vi "GTcode_v6(reorganized).vi"() -> ()   [LabVIEW 2016]
uses:
  DCScode_simulISS_MAP/flex05-4chPascal.dll
  <vilib>/Utility/config.llb/NI_LVConfig.lvlib
  <vilib>/Utility/config.llb/Write Key (U32).vi
  <vilib>/Utility/config.llb/Read Key (U32).vi
  DCScode_simulISS_MAP/flex05oem8chauto100nsPASCAL_win7.dll
  <vilib>/Analysis/NI_AALBase.lvlib
  <vilib>/Analysis/NI_AALPro.lvlib
  <vilib>/Utility/config.llb/Write Key (I32).vi
  <vilib>/Utility/config.llb/Write Key (Double).vi
  <vilib>/Utility/config.llb/Write Key (String).vi
  <vilib>/Utility/config.llb/Read Key (I32).vi
  <vilib>/Waveform/WDTOps.llb/WDT Append Waveforms DBL.vi
  <vilib>/Waveform/WDTFileIO.llb/ Write Waveform to File.vi
  <vilib>/Analysis/5stat.llb/RMS (DBL).vi
panel:
  in  "Tab\nControl":T1(tab)=enum."Real Time Fitting Parameters" caption="Tab Control"
  out "mean":dbl format="%0.1e"
  out "COV":dbl format="%0.1f"
  in  "Fixed Time":bool
  in  "Detector Used":T2(ring)=enum."Det 2"
  in  "Real Time Fitting?":bool=TRUE
  out "g2":cluster{"Delay Time":sgl[], sgl[]}[](graph) caption="Normalized Correlation Function"
  out "Tau":cluster{"tmp":dbl, dbl}(graph) caption="Relative Changes of Flow"
  in  "QUIT":bool
  in  "Clear plots":bool
  in  "Baseline":bool
  in  "MARK\nMark":bool
  in  "Stop":bool
  in  "Sequence Scan":bool
  out "Mark #":u32
  out "Trial #":u32
  out "Frame #":u32
  out "Det 8":sgl format="%.3f"
  out "Det 7":sgl format="%.3f"
  out "Det 6":sgl format="%.3f"
  out "Det 5":sgl format="%.3f"
  out "Det 4":sgl format="%.3f"
  out "Det 3":sgl format="%.3f"
  out "Det 2":sgl format="%.3f"
  out "Det 1":sgl format="%.3f"
  out "Computer Time":string="2010-1-12 23:16:10"
  in  "D1":bool
  in  "D2":bool
  in  "D3":bool
  in  "D4":bool
  in  "D5":bool
  in  "D6":bool
  in  "D7":bool
  in  "D8":bool
  out "Tau 2":T3(graph)={1.6593152555505744e-08, 3.9427894777554196e-08, 4.065716407938411e-08, 1.5135790977358522e-08, 2.4870420100428357e-08, 7.094765128107397e-08, 0.0, 4.1348620928852906e-07, 1.5886917674344795e-08, 4.0280526032721455e-08, -1.0, -1.0} caption="Blood Flow Index (cm2/s)"
  in  "Fixed # of Frames":u32=5
  out "Status":string="Quit"
  in  "Optical Switch OPEN":bool
  in  "Delay between frames(ms)":u32=500
  out "Time Left (ms)":sgl format="%.3f"
  in  "Integration Time (ms)":sgl=1000.0 min=1 max=13000 step=1
  in  "File Name:":string="test0"
  in  "Data Save Directory:":path=path "C:/data"
  in  "ISS Lasers ON":bool
  in  "Test":bool
  out "Moving Avg RMS":dbl(slide) scale=0.0..0.07
  out "raw data":dynamicdata(graph)
  out "Trial Data 2":waveform(dbl)(graph)
  out "Moving Avg RMS Graph":dbl(graph)
  out "Reset Data Acquisition\nAnd UI Updating":bool=TRUE
  out "Trial In Progress":bool
  in  "Lines":tag="Dev1/port1/line0:1, Dev1/port1/line3:7"
  in  "Delaytime(ms)":u32=200
  in  "Initialize Correlator":bool
  in  "Detector Select":enum32{"4 Detectors", "8 Detectors"}(radio)=enum."8 Detectors"
  in  "Update Time (ms)\nDO NOT CHANGE!":u32=105 min=1 max=999 step=1
  in  "Laser Input Name":refnum<visa-resource-name>="COM7"
  out "Flow in each detector":dbl[](array[numeric])=[-1.0, -1.0, -1.0, -1.0, -1.0, -1.0, -1.0, -1.0, -1.0, -1.0, -1.0, -1.0]
  in  "Visible\nAverages":bool[](array[boolean])=[FALSE, FALSE, FALSE, FALSE]
  in  "Avg":bool[][](array[boolean])=[[FALSE, FALSE, FALSE, FALSE, FALSE, FALSE, FALSE, FALSE], [FALSE, FALSE, FALSE, FALSE, FALSE, FALSE, FALSE, FALSE], [FALSE, FALSE, FALSE, FALSE, FALSE, FALSE, FALSE, FALSE], [FALSE, FALSE, FALSE, FALSE, FALSE, FALSE, FALSE, FALSE]]
  in  "rho":dbl[](array[numeric])=[2.5, 2.5, 2.5, 2.5, 2.5, 2.5, 2.5, 2.5, -1.0, -1.0, -1.0, -1.0]
  in  "Other Settings":u32[](array[numeric])=[1, 120, 0, 1] caption="Flow in each detector"
  in  "Initial Guess":dbl[](array[numeric])=[1e-08, 0.5, 0.05, 10.0] caption="Flow in each detector"
  in  "Lower Cut-Off":dbl=20.0
  in  "Upper Cut-Off (Not In Use)":dbl=300.0 caption="Upper Cut-Off"
  in  "Sample rate (Hz)":dbl=22050.0
  in  "Frames Per Second":dbl
  in  "Moving Average Length (s)":dbl
  in  "VR Data Input File":path
  in  "VR Percent Path":path
  out "Bufffer Index":dbl
  out "Frames in Buffer":dbl
  out "Samples per frame":dbl
  out "Filtered data":waveform(dbl)
  out "Rectified Moving Average Sample":waveform(dbl)[](graph)
  out "Trial Data":waveform(dbl)
  in  "Trial Number":dbl
  in  "Target Percentage":dbl
  out "Aggregate Data":waveform(dbl)[](array[waveform])
  out "4CH?":bool
  out "Detector#":u32=1
  out "Source#":u32=1
  # "kHz"
  # "kHz"
  # "Don't Change these Parameters unless you know clearly what you are doing"
  # "ISS Triggers Setup"
  # "Channel Parameters"
  # "Step1"
  # "Line"
  # "0"
  # "1"
  # "3"
  # "4"
  # "5"
  # "6"
  # "7"
  # "*The number of lines in the list must\nmatch the number of elements in\nthe array."
  # "Step2"
  # "Line"
  # "0"
  # "1"
  # "3"
  # "4"
  # "5"
  # "6"
  # "7"
  # "Step3"
  # "Line"
  # "0"
  # "1"
  # "3"
  # "4"
  # "5"
  # "6"
  # "7"
  # "Line    Signal\n\n0           ISS Trigger (0: OFF, 1: ON)\n1           Flow Laser 1 ON/OFF (0:OFF, 1:ON)\n2           ISS Data Acquisition (0: DONE, 1: NO)\n3           ISS Laser ON/OFF (0: ON, 1: OFF)\n4           Trigger for Marks  (0: OFF, 1: ON)\n5           Flow Laser 2 ON/OFF (0:OFF, 1:ON)\n6           Reserved\n7           Reserved"
  # "Wait ISS Data Acuisition DONE Signal"
  # "Step4"
  # "Step5"
  # "Line"
  # "0"
  # "1"
  # "3"
  # "4"
  # "5"
  # "6"
  # "7"
  # "Flow Lasers Setup"
  # "FROM FRONT PANEL"
  # "Line"
  # "0"
  # "1"
  # "3"
  # "4"
  # "5"
  # "6"
  # "7"
  # "Line"
  # "0"
  # "1"
  # "3"
  # "4"
  # "5"
  # "6"
  # "7"
  # "Det 1"
  # "Det 2"
  # "Det 3"
  # "Det 4"
  # "Det 5"
  # "Det 6"
  # "Det 7"
  # "Det 8"
  # "Avg 1"
  # "Avg 2"
  # "Avg 3"
  # "Avg 4"
  # "Db"
  # "Beta"
  # "Mua"
  # "MuS'"
  # "1"
  # "2"
  # "3"
  # "4"
  # "5"
  # "6"
  # "7"
  # "8"
  # "Avg 1"
  # "Starting Pt"
  # "End Pt"
  # "Approximate"
  # "Variables"
  # "Avg 2"
  # "Avg 3"
  # "Avg 4"
  # "Source Detector  Separations"
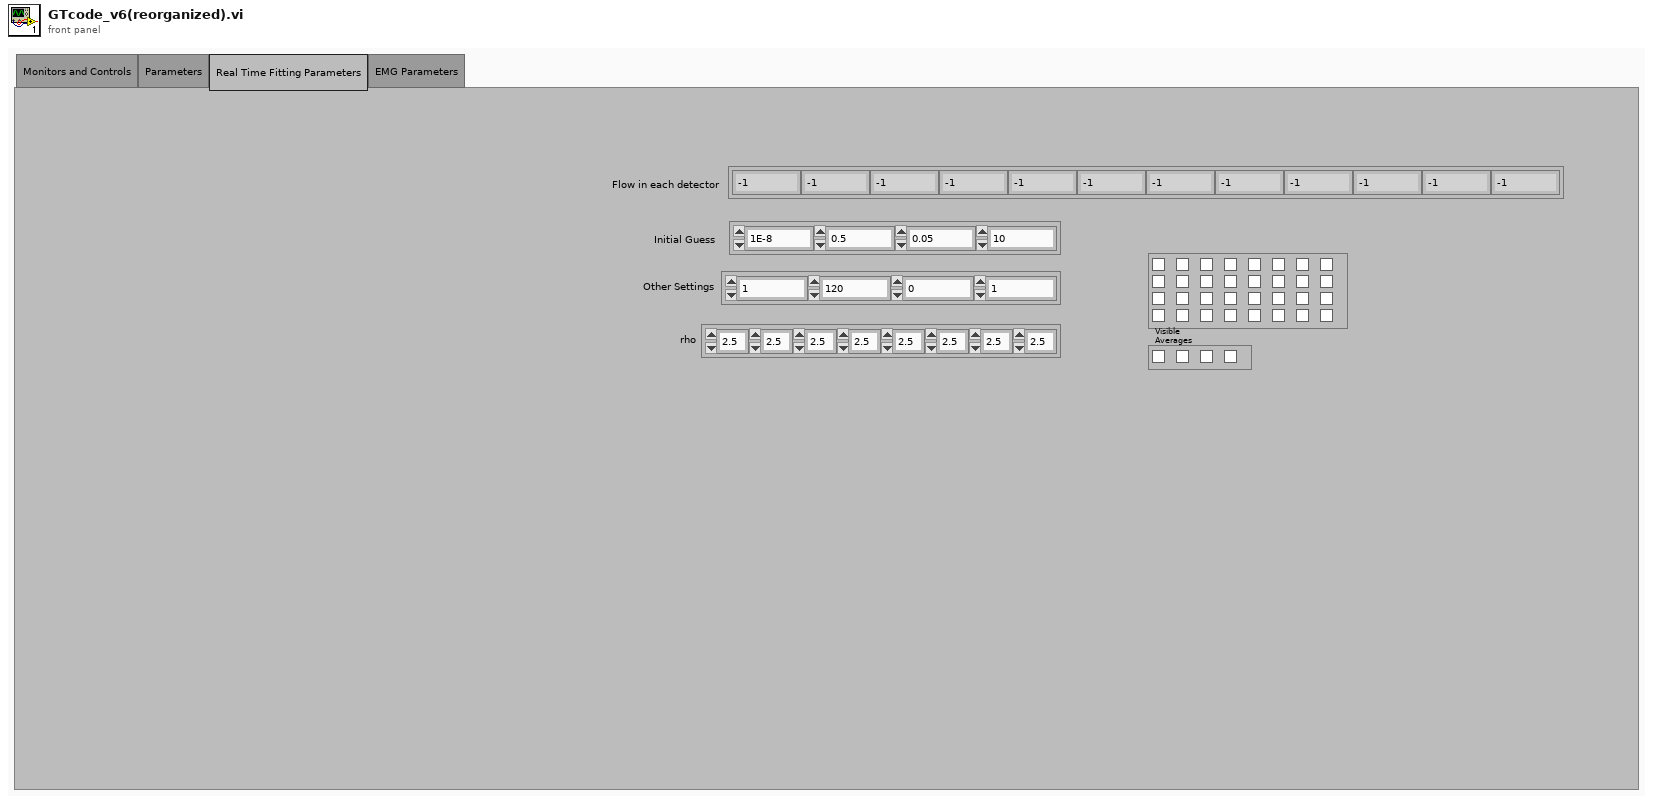
[diagram p1: front panel]
types:
  T1 = enum32{"Monitors and Controls", "Parameters", "Real Time Fitting Parameters", "EMG Parameters"}
  T2 = enum16{"Det 1", "Det 2", "Det 3", "Det 4", "Det 5", "Det 6", "Det 7", "Det 8"}
  T3 = cluster{dbl, dbl, dbl, dbl, dbl, dbl, dbl, dbl, dbl, dbl, dbl, dbl}
  T4 = typedef "WaveformArrayControl.ctl" = waveform(dbl)[]
  T5 = enum8{"Enabled", "Disabled", "Disabled and Grayed Out"}
  T6 = cluster{dbl, dbl, dbl, dbl, dbl, dbl, dbl, dbl, dbl, dbl, dbl, dbl}[]
  T7 = typedef "NI_LVConfig.lvlib/Config Data RefNum.ctl" = refnum<k1>
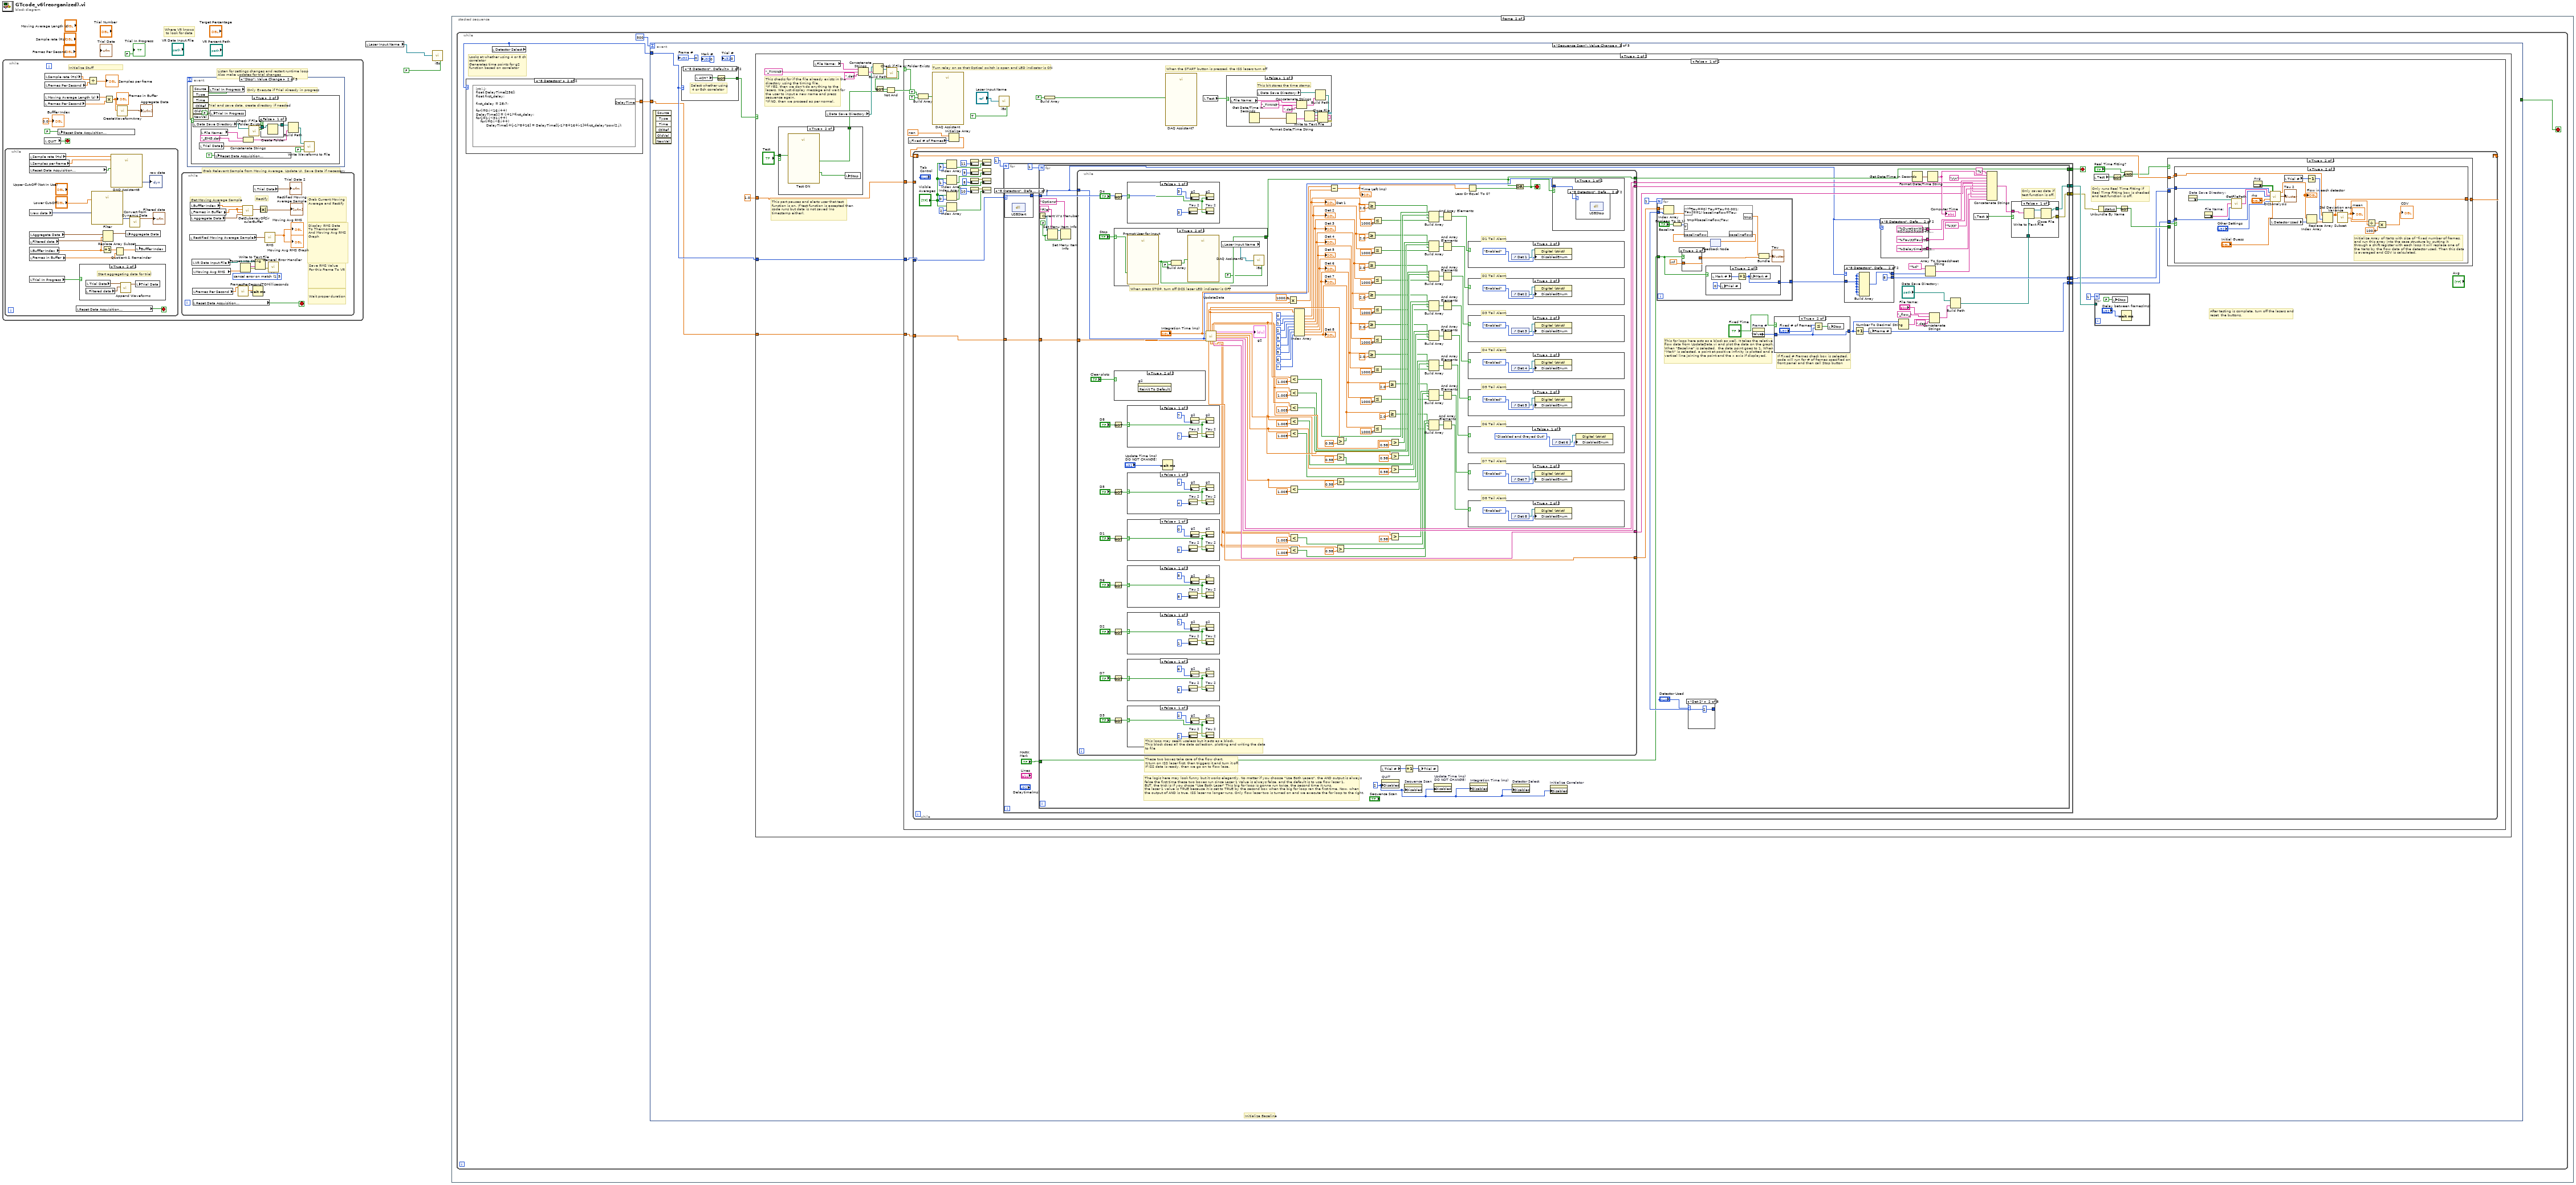
[diagram p0: block diagram]
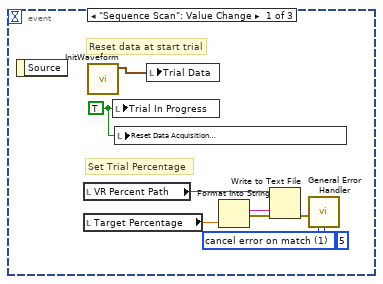
[diagram p2: hidden frame]
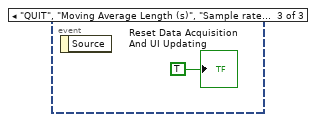
[diagram p5: hidden frame]
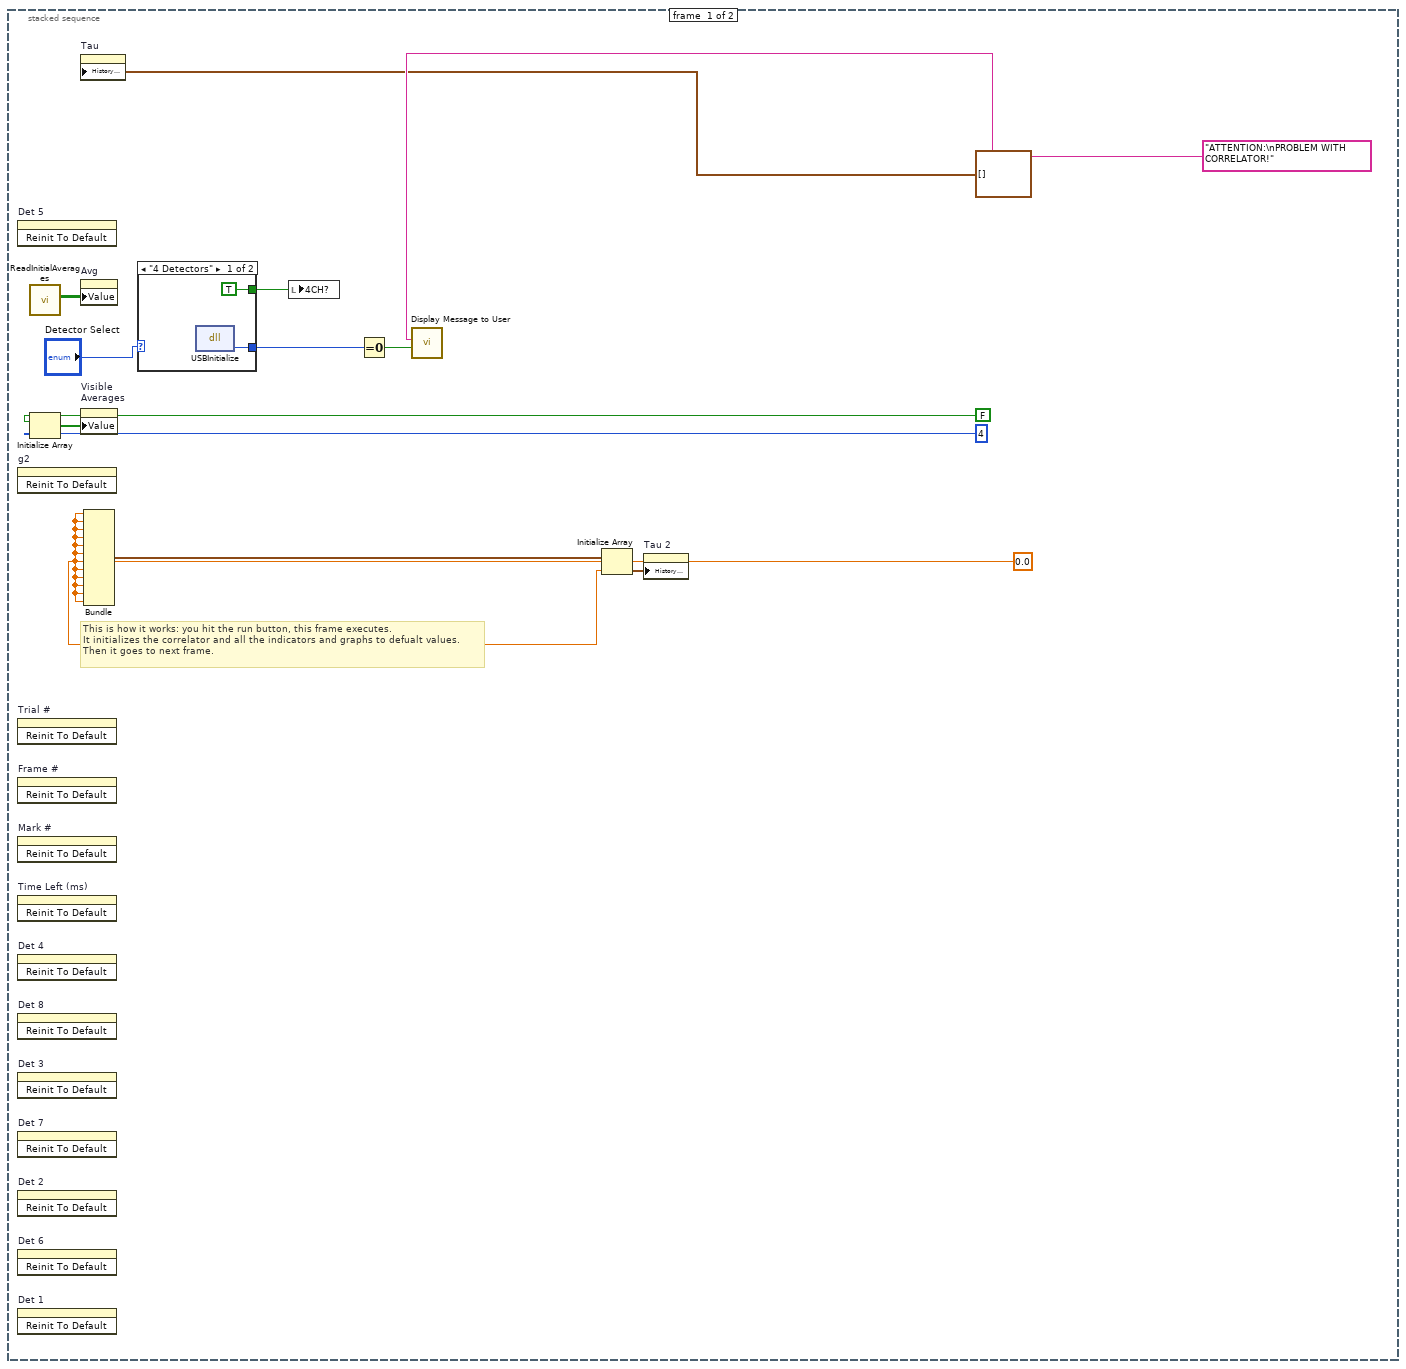
[diagram p7: hidden frame]
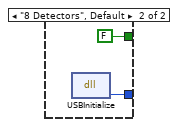
[diagram p8: hidden frame]
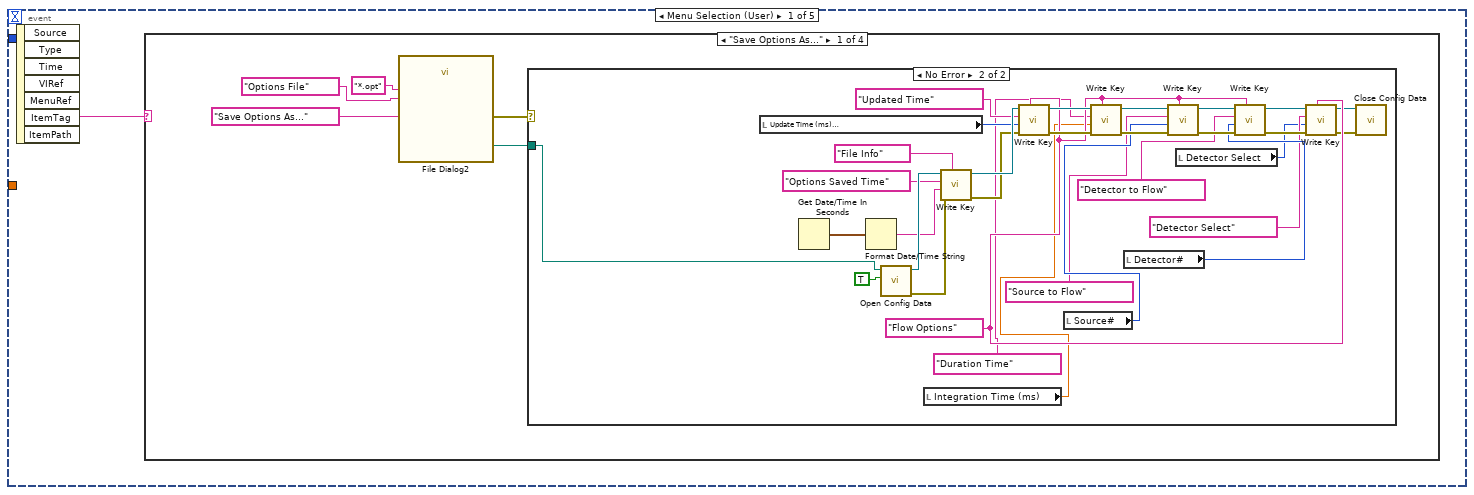
[diagram p10: hidden frame]
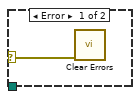
[diagram p11: hidden frame]
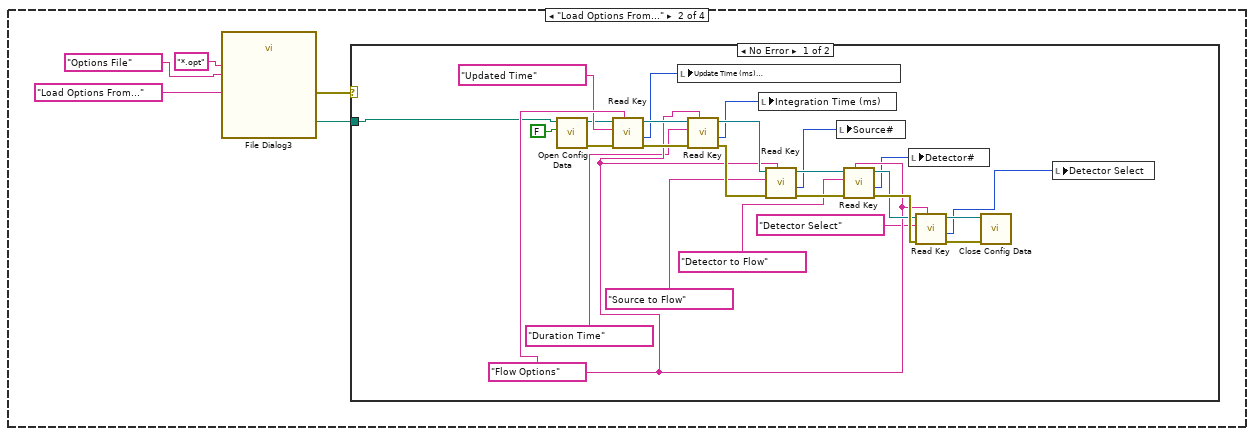
[diagram p12: hidden frame]
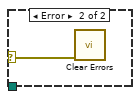
[diagram p13: hidden frame]
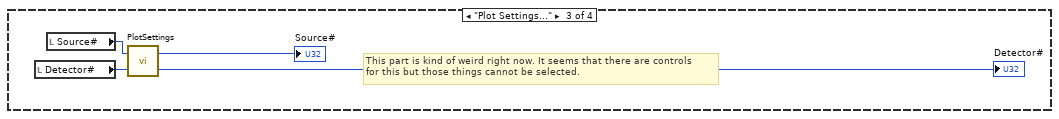
[diagram p14: hidden frame]
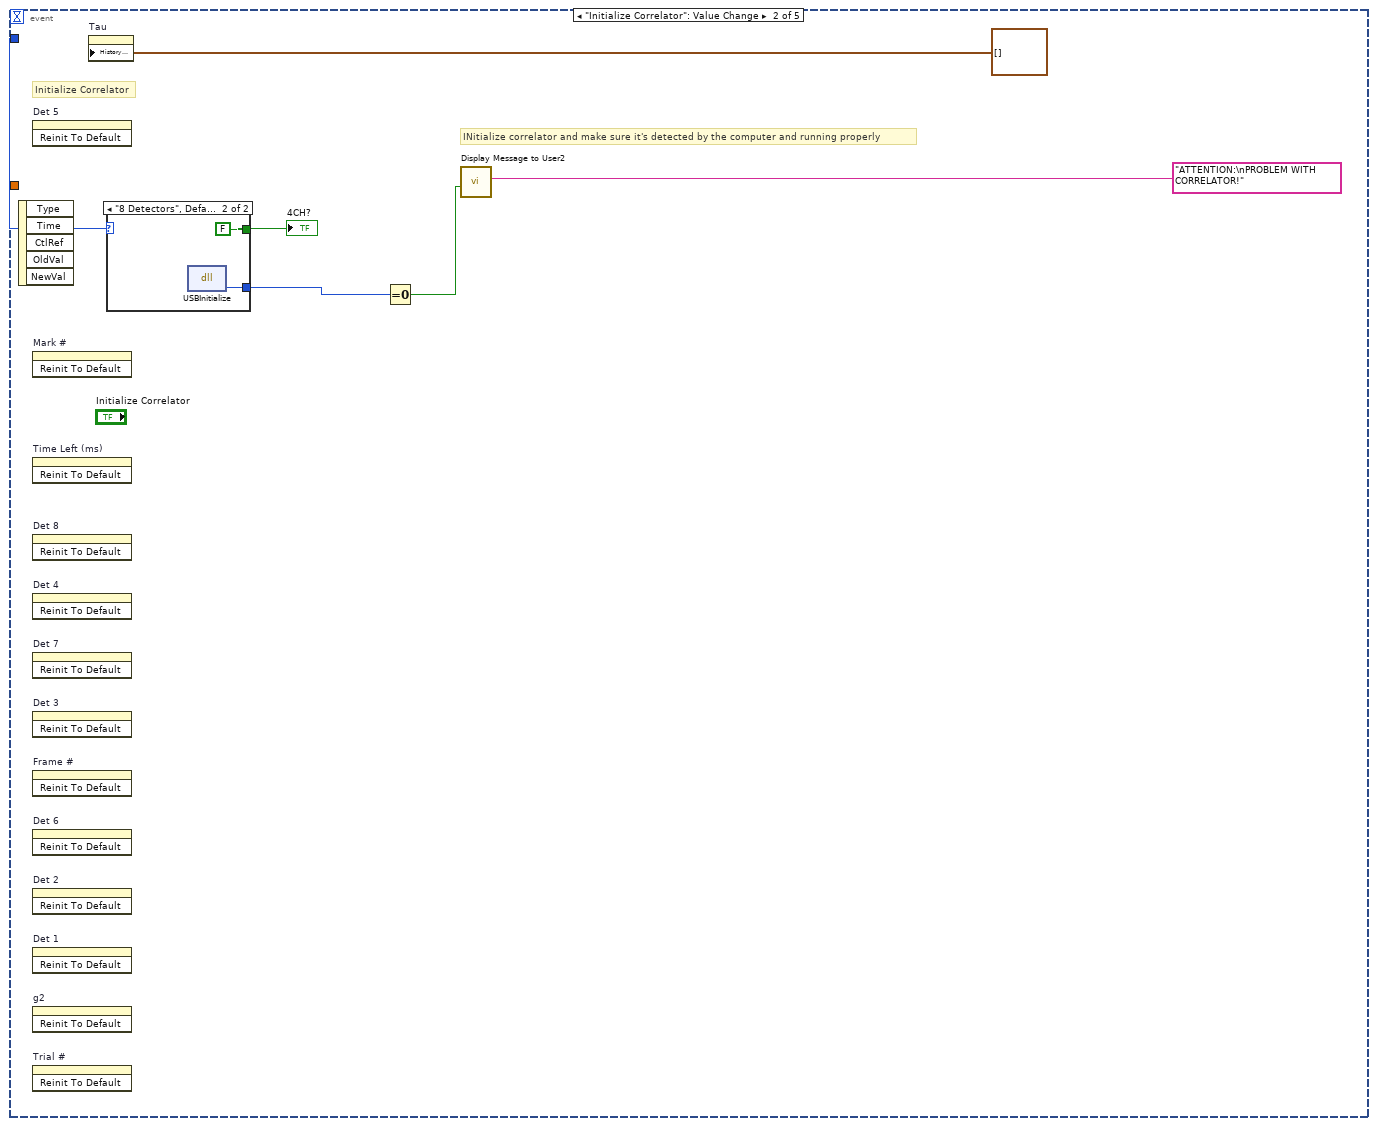
[diagram p16: hidden frame]
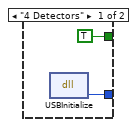
[diagram p17: hidden frame]
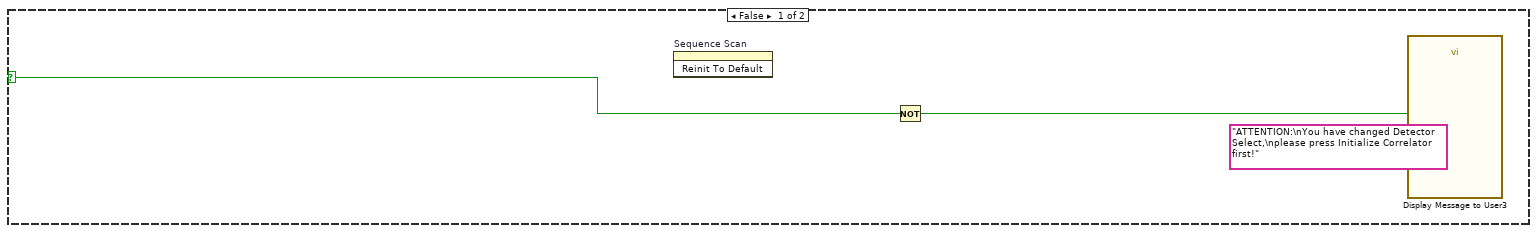
[diagram p18: hidden frame]
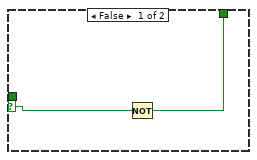
[diagram p19: hidden frame]
diagram:
  # "Where VR knows\n to look for data"
  n1 = while {
    stop <- w4 stop-if-true
    # "Grab Relevant Sample from Moving Average, Update UI, Save Data if necessary"
    # "Initialize Stuff"
    # "Listen for settings changes and restart runtime loop\nAlso make updates for trial changes"
    n2 = while {
      stop <- w60 stop-if-true
      n3 = local read "Sample rate (Hz)"() -> (w74:dbl)
      n4 = local read "Samples per frame"() -> (w73:dbl)
      n5 = local read "Reset Data Acquisition\nAnd UI Updating"() -> (w59:bool)
      n6 = local read "raw data"() -> (w71:dynamicdata)
      n7 = local read "Aggregate Data"() -> (w67:waveform(dbl)[])
      n8 = local read "Filtered data"() -> (w66:waveform(dbl))
      n9 = local read "Bufffer Index"() -> (w65:dbl)
      n10 = local read "Frames in Buffer"() -> (w62:dbl)
      n11 = local read "Trial In Progress"() -> (w58:bool)
      n12 = local read "Reset Data Acquisition\nAnd UI Updating"() -> (w60:bool)
      n13 = case shown="True" w58 {
        frame False {
        }
        frame True {
          # "Start aggregating data for trial"
          n14 = local read "Filtered data"() -> (w76:waveform(dbl))
          n15 = local read "Trial Data"() -> (w77:waveform(dbl))
          n16 = call-poly <vilib>:"Append Waveforms.vi"("waveform B"=w76, "waveform A"=w77) -> ("waveform out"=w75:waveform(dbl))  [unwired: 8 in, 1 out]
          n17 = local write "Trial Data"(w75) -> ()
        }
      }
      n18 = call "Filter"("Lower Cut-Off"="Lower Cut-Off", "Signal"=w71) -> ("Filtered Signal"=w69:dynamicdata)  [unwired: 8 in, 1 out]
      n19 = Increment(x=w65) -> (x+1=w61:dbl)
      n20 = Replace Array Subset(array=w67, new element=w66, index=w65) -> (w64:waveform(dbl)[])
      n21 = call "DAQ Assistant8"("rate"=w74, "number of samples"=w73, "stop (T)"=w59) -> ("data"=→"raw data":dynamicdata)  [unwired: 14 in, 2 out]
      n22 = Quotient & Remainder(x=w61, y=w62) -> (x-y*floor(x/y)=w63:dbl)  [unwired: 1 out]
      n23 = local write "Aggregate Data"(w64) -> ()
      n24 = call "Convert from Dynamic Data"("Dynamic Data Type"=w69) -> ("Waveform"=→"Filtered data":waveform(dbl))  [unwired: 3 in]
      n25 = local write "Bufffer Index"(w63) -> ()
    }
    n26 = local read "Moving Average Length (s)"() -> (w10:dbl)
    n27 = local read "Frames Per Second"() -> (w9:dbl)
    n28 = local read "QUIT"() -> (w4:bool)
    n29 = local read "Sample rate (Hz)"() -> (w13:dbl)
    n30 = local read "Frames Per Second"() -> (w12:dbl)
    n31 = local write "Reset Data Acquisition\nAnd UI Updating"(FALSE) -> ()
    n32 = Divide(x=w13, y=w12) -> (x/y=→"Samples per frame":dbl)
    n33 = Multiply(x=w10, y=w9) -> (x*y=w5:dbl)
    "Frames in Buffer" <- w5
    n34 = call "CreateWaveformArray.vi"("bufferSize"=w5) -> ("initialized array"=→"Aggregate Data":waveform(dbl)[])  [unwired: 5 in, 1 out]
    n35 = while {
      stop <- w57 stop-if-true
      w47 = 1 items=["no exception", "cancel error on match", "set error on match"] ("[exception action] (none:0)")
      # "Wait proper duration"
      # "Save RMS Value\nFor this Frame To VR"
      # "Display RMS Data\nTo Thermometer\nAnd Moving Avg RMS\nGraph"
      # "Grab Current Moving\nAverage and Rectify"
      # "Get Moving Average Sample"
      # "Rectify"
      n36 = local read "Rectified Moving Average Sample"() -> (w50:waveform(dbl)[])
      n37 = local read "Bufffer Index"() -> (w56:dbl)
      n38 = local read "Frames in Buffer"() -> (w55:dbl)
      n39 = local read "Aggregate Data"() -> (w54:waveform(dbl)[])
      n40 = local read "VR Data Input File"() -> (w43:path)
      n41 = local read "Moving Avg RMS"() -> (w41:dbl)
      n42 = local read "Frames Per Second"() -> (w49:dbl)
      n43 = local read "Reset Data Acquisition\nAnd UI Updating"() -> (w57:bool)
      n44 = call "FramesPerSecondTOMilliseconds.vi"("Thermometer\nFps"=w49) -> ("x*y"=w48:dbl)  [unwired: 10 in]
      n45 = Format Into String(w41) -> (resulting string=w42:string, error out=w44:errorcluster)  [unwired: 3 in]
      n46 = call "GetSubarrayOfCircularBuffer.vi"("initialized array"=w54, "buffer size"=w55, "subset size"=w55, "start index"=w56) -> ("initialized array 2"=w53:T4)  [unwired: 7 in]
      n47 = Wait (ms)(milliseconds to wait=w48) -> ()  [unwired: 1 out]
      n48 = local read "Trial Data"() -> (→"Trial Data 2":waveform(dbl))
      n49 = Write to Text File(file (use dialog)=w43, text=w42, error in=w44) -> (error out=w45:errorcluster)  [unwired: 1 in, 2 out]
      n50 = Absolute Value(x=w53) -> (abs(x)=→"Rectified Moving Average Sample":T4)
      n51 = call-poly <vilib>:"RMS.vi"("X"=w50) -> ("rms value"=→"Moving Avg RMS" →"Moving Avg RMS Graph":dbl)  [unwired: 1 out]
      n52 = call <vilib>:"General Error Handler.vi"("error in (no error)"=w45, "[exception action] (none:0)"=w47, "[exception code]"=5) -> ()  [unwired: 8 in, 5 out]
    }
    n53 = event shown="[1] \"Stop\": Value Change" {
      selector: _ -> [_ _ _]
      dyn-events: _ -> [_ _ _]
      timeout: _ -> [_ _ _]
      event "Sequence Scan": Value Change {
        w20 = 1 items=["no exception", "cancel error on match", "set error on match"] ("[exception action] (none:0)")
        w21 = TRUE ("Trial In Progress")
        # "Set Trial Percentage"
        # "Reset data at start trial"
        n54 = event-data() -> ()  [unwired: 1 in, 1 out]
        n55 = local read "VR Percent Path"() -> (w15:path)
        n56 = local read "Target Percentage"() -> (w14:dbl)
        n57 = call "InitWaveform.vi"() -> ("output waveform"=w22:waveform(dbl))  [unwired: 11 in]
        n58 = local write "Trial In Progress"(w21) -> ()
        n59 = local write "Reset Data Acquisition\nAnd UI Updating"(w21) -> ()
        n60 = local write "Trial Data"(w22) -> ()
        n61 = Format Into String(w14) -> (resulting string=w16:string, error out=w17:errorcluster)  [unwired: 3 in]
        n62 = Write to Text File(file (use dialog)=w15, text=w16, error in=w17) -> (error out=w18:errorcluster)  [unwired: 1 in, 2 out]
        n63 = call <vilib>:"General Error Handler.vi"("error in (no error)"=w18, "[exception action] (none:0)"=w20, "[exception code]"=5) -> ()  [unwired: 8 in, 5 out]
      }
      event "Stop": Value Change {
        # "Only Execute if Trial Already in progress"
        n64 = event-data() -> ()  [unwired: 1 in, 6 out]
        n65 = local read "Trial In Progress"() -> (w23:bool)
        n66 = case shown="True" w23 {
          frame False {
          }
          frame True {
            # "End Trial and save data, create directory if needed"
            n67 = local read "Data Save Directory:"() -> (w27:path)
            n68 = local read "Trial Data"() -> (w34:waveform(dbl))
            n69 = local read "File Name:"() -> (w26:string)
            n70 = local write "Trial In Progress"(FALSE ("Trial In Progress")) -> ()
            n71 = local write "Reset Data Acquisition\nAnd UI Updating"(TRUE ("Reset Data Acquisition\nAnd UI Updating")) -> ()
            n72 = Concatenate Strings(w26, "_EMG.dat" ("string")) -> (w24:string)
            n73 = call <vilib>:"Check if File or Folder Exists.vi"("path"=w27) -> ("file or folder exists?"=w31:bool, "dup path"=w29:path)  [unwired: 8 in, 1 out]
            n74 = case shown="False" w31 {
              tunnel: [w36 w38] -> w30
              tunnel: w29 -> [w37 w38]
              frame False {
                n75 = Create Folder(path (use dialog)=w37) -> (created path=w36:path)  [unwired: 2 in, 2 out]
              }
              frame True {
              }
            }
            n76 = Build Path(base path=w30, name or relative path=w24) -> (appended path=w28:path)
            n77 = call-poly <vilib>:"Write Waveforms to File.vi"("append to file? (new file:F)"=FALSE, "waveform"=w34, "file path (dialog if empty)"=w28) -> ()  [unwired: 7 in, 2 out]
          }
        }
      }
      event "QUIT", "Moving Average Length (s)", "Sample rate (Hz)", "Frames Per Second": Value Change {
        n78 = event-data() -> ()  [unwired: 1 in, 1 out]
        "Reset Data Acquisition\nAnd UI Updating" <- TRUE
      }
    }
    "Bufffer Index" <- 0.0 ("Bufffer Index")
  }
  n79 = local read "Laser Input Name"() -> (w2:refnum<visa-resource-name>)
  n80 = call "iBs.vi"("Laser On/Off"=FALSE, "VISA resource name"=w2) -> ()
  n81 = stacked-sequence {
    frame #0 {
      w80 = 0.0
      # "This is how it works: you hit the run button, this frame executes.\nIt initializes the correlator and all the indicators and graphs to defualt values.\nThen it goes to next frame."
      n82 = invoke on="Det 5" class="DigNum (strict)" method="Reinit To Default"() -> ()  [unwired: 3 in, 3 out]
      n83 = invoke on="g2" class="XYGraph (strict)" method="Reinit To Default"() -> ()  [unwired: 3 in, 3 out]
      n84 = invoke on="Trial #" class="DigNum (strict)" method="Reinit To Default"() -> ()  [unwired: 3 in, 3 out]
      n85 = invoke on="Frame #" class="DigNum (strict)" method="Reinit To Default"() -> ()  [unwired: 3 in, 3 out]
      n86 = invoke on="Mark #" class="DigNum (strict)" method="Reinit To Default"() -> ()  [unwired: 3 in, 3 out]
      n87 = invoke on="Time Left (ms)" class="DigNum (strict)" method="Reinit To Default"() -> ()  [unwired: 3 in, 3 out]
      n88 = invoke on="Det 4" class="DigNum (strict)" method="Reinit To Default"() -> ()  [unwired: 3 in, 3 out]
      n89 = invoke on="Det 8" class="DigNum (strict)" method="Reinit To Default"() -> ()  [unwired: 3 in, 3 out]
      n90 = invoke on="Det 3" class="DigNum (strict)" method="Reinit To Default"() -> ()  [unwired: 3 in, 3 out]
      n91 = invoke on="Det 7" class="DigNum (strict)" method="Reinit To Default"() -> ()  [unwired: 3 in, 3 out]
      n92 = invoke on="Det 2" class="DigNum (strict)" method="Reinit To Default"() -> ()  [unwired: 3 in, 3 out]
      n93 = invoke on="Det 6" class="DigNum (strict)" method="Reinit To Default"() -> ()  [unwired: 3 in, 3 out]
      n94 = invoke on="Det 1" class="DigNum (strict)" method="Reinit To Default"() -> ()  [unwired: 3 in, 3 out]
      n95 = call "ReadInitialAverages.vi"() -> ("avgOut"=w79:bool[][])  [unwired: 11 in]
      n96 = Initialize Array(FALSE, 4) -> (w78:bool[])
      n97 = property on="Tau" class="WFChart (strict)"("History Data"=cluster{"tmp":dbl, dbl}[] []) -> ()  [unwired: 2 in, 2 out]
      n98 = property on="Avg" class="Arr (strict)"("Value"=w79) -> ()  [unwired: 2 in, 2 out]
      n99 = property on="Visible\nAverages" class="Arr (strict)"("Value"=w78) -> ()  [unwired: 2 in, 2 out]
      n100 = Bundle(w80, w80, w80, w80, w80, w80, w80, w80, w80, w80, w80, w80) -> (w82:T3)  [unwired: 1 in]
      n101 = case shown="\"4 Detectors\"" "Detector Select" {
        tunnel: [w92 w94] -> w90
        tunnel: [TRUE FALSE] -> w88
        frame "4 Detectors" {
          n102 = dll-call lib="C:/Users/BUCKLEY-ADMIN/Desktop/DCScode_simulISS_MAP/flex05-4chPascal.dll" fn="USBInitialize" label="InitCH4"() -> ("return type"=w92:u8)  [unwired: 3 in, 2 out]
        }
        frame "8 Detectors", Default {
          n103 = dll-call lib="C:/Users/BUCKLEY-ADMIN/Desktop/DCScode_simulISS_MAP/flex05oem8chauto100nsPASCAL_win7.dll" fn="USBInitialize" label="InitCH8"() -> ("return type"=w94:u8)  [unwired: 3 in, 2 out]
        }
      }
      n104 = local write "4CH?"(w88) -> ()
      n105 = Equal To 0?(x=w90) -> (x = 0?=w89:bool)
      n106 = call "Display Message to User"("Enable"=w89, "Message"="ATTENTION:\nPROBLEM WITH CORRELATOR!") -> ()  [unwired: 8 in, 2 out]
      n107 = Initialize Array(w82, w80) -> (w81:T6)
      n108 = property on="Tau 2" class="WFChart (strict)"("History Data"=w81) -> ()  [unwired: 2 in, 2 out]
    }
    frame #1 {
      n109 = while {
        stop <- w95 stop-if-true
        # "Looks at whether using 4 or 8 ch correlator\nGenerates time points for g2 function based on correlator"
        n110 = local read "Detector Select"() -> (w96:enum32{"4 Detectors", "8 Detectors"})
        n111 = case shown="\"8 Detectors\"" w96 {
          tunnel: [_ w99] -> w97
          frame "4 Detectors", Default {
          }
          frame "8 Detectors" {
            n112 = formula code="int i,j;\nfloat DelayTime[256];\nfloat first_delay;\n\nfirst_delay = 2E-7;\n\nfor(i=0;i<16;i++)\nDelayTime[i] = (i+1)*first_delay;\nfor(j=1;j<31;j++)\n    for(i=0;i<8;i++)\n         DelayTime[i+(j-1)*8+16] = DelayTime[(j-1)*8+16+i-1]+first_delay*pow(2,j);"() -> ("DelayTime"=w99:dbl[])
          }
        }
        n113 = event shown="[2] \"Sequence Scan\": Value Change" {
          selector: _ -> [_ _ _ _ _]
          dyn-events: _ -> [_ _ _ _ _]
          timeout: 500 -> [_ _ _ _ _]
          tunnel: w97 -> [_ _ w184 _ _]
          tunnel: [_ _ _ "QUIT" _] -> w95
          tunnel: w96 -> [_ w176 w185 w674 _]
          event Menu Selection (User) {
            n114 = event-data() -> ("ItemTag"=w100:string)  [unwired: 1 in, 6 out]
            n115 = case shown="\"Save Options As...\"" w100 {
              frame "Save Options As..." {
                n116 = call "File Dialog2"("prompt"="Save Options As...", "pattern (all files)"="*.opt", "pattern label"="Options File") -> ("selected path"=w102:path, "error out"=w101:errorcluster)  [unwired: 9 in, 2 out]
                n117 = case shown="No Error" w101 {
                  selector: w101 -> [w106 _]
                  tunnel: w102 -> [_ w137]
                  frame Error {
                    n118 = call <vilib>:"Clear Errors.vi"("error in (no error)"=w106) -> ()  [unwired: 5 in, 2 out]
                  }
                  frame No Error {
                    w124 = "Flow Options"
                    n119 = local read "Update Time (ms)\nDO NOT CHANGE!"() -> (w117:u32)
                    n120 = Get Date/Time In Seconds() -> (seconds since 1Jan1904=w123:timestamp)
                    n121 = Format Date/Time String(seconds (now)=w123) -> (date/time string=w119:string)  [unwired: 2 in]
                    n122 = call <vilib>:"Open Config Data.vi"("create file if necessary (T)"=TRUE, "configuration file path"=w137) -> ("error out"=w135:errorcluster, "refnum"=w134:T7)  [unwired: 7 in, 1 out]
                    n123 = local read "Integration Time (ms)"() -> (w115:sgl)
                    n124 = call-poly <vilib>:"Write Key.vi"("section"="File Info", "error in (no error)"=w135, "value"=w119, "key"="Options Saved Time", "refnum"=w134) -> ("error out"=w121:errorcluster, "refnum out"=w122:T7)  [unwired: 4 in, 1 out]
                    n125 = call-poly <vilib>:"Write Key.vi"("section"=w124, "error in (no error)"=w121, "value"=w117, "key"="Updated Time", "refnum"=w122) -> ("error out"=w133:errorcluster, "refnum out"=w132:T7)  [unwired: 4 in, 1 out]
                    n126 = local read "Source#"() -> (w114:u32)
                    n127 = call-poly <vilib>:"Write Key.vi"("section"=w124, "error in (no error)"=w133, "value"=w115, "key"="Duration Time", "refnum"=w132) -> ("error out"=w128:errorcluster, "refnum out"=w129:T7)  [unwired: 4 in, 1 out]
                    n128 = local read "Detector#"() -> (w111:u32)
                    n129 = call-poly <vilib>:"Write Key.vi"("section"=w124, "error in (no error)"=w128, "value"=w114, "key"="Source to Flow", "refnum"=w129) -> ("error out"=w130:errorcluster, "refnum out"=w131:T7)  [unwired: 4 in, 1 out]
                    n130 = local read "Detector Select"() -> (w109:enum32{"4 Detectors", "8 Detectors"})
                    n131 = call-poly <vilib>:"Write Key.vi"("section"=w124, "error in (no error)"=w130, "value"=w111, "key"="Detector to Flow", "refnum"=w131) -> ("error out"=w127:errorcluster, "refnum out"=w126:T7)  [unwired: 4 in, 1 out]
                    n132 = call-poly <vilib>:"Write Key.vi"("section"=w124, "error in (no error)"=w127, "value"=w109, "key"="Detector Select", "refnum"=w126) -> ("error out"=w107:errorcluster, "refnum out"=w108:T7)  [unwired: 4 in, 1 out]
                    n133 = call <vilib>:"Close Config Data.vi"("error in (no error)"=w107, "refnum"=w108) -> ()  [unwired: 8 in, 2 out]
                  }
                }
              }
              frame "Load Options From..." {
                n134 = call "File Dialog3"("prompt"="Load Options From...", "pattern (all files)"="*.opt", "pattern label"="Options File") -> ("selected path"=w139:path, "error out"=w138:errorcluster)  [unwired: 9 in, 2 out]
                n135 = case shown="No Error" w138 {
                  selector: w138 -> [_ w168]
                  tunnel: w139 -> [w143 _]
                  frame No Error {
                    w158 = "Flow Options"
                    n136 = call <vilib>:"Open Config Data.vi"("create file if necessary (T)"=FALSE, "configuration file path"=w143) -> ("error out"=w150:errorcluster, "refnum"=w149:T7)  [unwired: 7 in, 1 out]
                    n137 = call-poly <vilib>:"Read Key.vi"("section"=w158, "error in (no error)"=w150, "key"="Updated Time", "refnum"=w149) -> ("error out"=w166:errorcluster, "value"=w148:u32, "refnum out"=w165:T7)  [unwired: 4 in, 1 out]
                    n138 = local write "Update Time (ms)\nDO NOT CHANGE!"(w148) -> ()
                    n139 = call-poly <vilib>:"Read Key.vi"("section"=w158, "error in (no error)"=w166, "key"="Duration Time", "refnum"=w165) -> ("error out"=w161:errorcluster, "value"=w147:i32, "refnum out"=w162:T7)  [unwired: 4 in, 1 out]
                    n140 = local write "Integration Time (ms)"(w147) -> ()
                    n141 = call-poly <vilib>:"Read Key.vi"("section"=w158, "error in (no error)"=w161, "key"="Source to Flow", "refnum"=w162) -> ("error out"=w163:errorcluster, "value"=w144:u32, "refnum out"=w164:T7)  [unwired: 4 in, 1 out]
                    n142 = local write "Source#"(w144) -> ()
                    n143 = call-poly <vilib>:"Read Key.vi"("section"=w158, "error in (no error)"=w163, "key"="Detector to Flow", "refnum"=w164) -> ("error out"=w160:errorcluster, "value"=w145:u32, "refnum out"=w159:T7)  [unwired: 4 in, 1 out]
                    n144 = local write "Detector#"(w145) -> ()
                    n145 = call-poly <vilib>:"Read Key.vi"("section"=w158, "error in (no error)"=w160, "key"="Detector Select", "refnum"=w159) -> ("error out"=w151:errorcluster, "value"=w146:u32, "refnum out"=w152:T7)  [unwired: 4 in, 1 out]
                    n146 = call <vilib>:"Close Config Data.vi"("error in (no error)"=w151, "refnum"=w152) -> ()  [unwired: 8 in, 2 out]
                    n147 = local write "Detector Select"(w146) -> ()
                  }
                  frame Error {
                    n148 = call <vilib>:"Clear Errors.vi"("error in (no error)"=w168) -> ()  [unwired: 5 in, 2 out]
                  }
                }
              }
              frame "Plot Settings..." {
                # "This part is kind of weird right now. It seems that there are controls\nfor this but those things cannot be selected."
                n149 = local read "Detector#"() -> (w170:u32)
                n150 = local read "Source#"() -> (w171:u32)
                n151 = call "PlotSettings.vi"("Detectorin"=w170, "Sourcein"=w171) -> ("Detector#"=→"Detector#":u32, "Source#"=→"Source#":u32)
              }
              frame Default {
              }
            }
          }
          event "Initialize Correlator": Value Change {
            # "INitialize correlator and make sure it's detected by the computer and running properly"
            # "Initialize Correlator"
            n152 = event-data() -> ()  [unwired: 1 in, 5 out]
            n153 = invoke on="Det 5" class="DigNum (strict)" method="Reinit To Default"() -> ()  [unwired: 3 in, 3 out]
            n154 = invoke on="Mark #" class="DigNum (strict)" method="Reinit To Default"() -> ()  [unwired: 3 in, 3 out]
            n155 = invoke on="Time Left (ms)" class="DigNum (strict)" method="Reinit To Default"() -> ()  [unwired: 3 in, 3 out]
            n156 = invoke on="Det 8" class="DigNum (strict)" method="Reinit To Default"() -> ()  [unwired: 3 in, 3 out]
            n157 = invoke on="Det 4" class="DigNum (strict)" method="Reinit To Default"() -> ()  [unwired: 3 in, 3 out]
            n158 = invoke on="Det 7" class="DigNum (strict)" method="Reinit To Default"() -> ()  [unwired: 3 in, 3 out]
            n159 = invoke on="Det 3" class="DigNum (strict)" method="Reinit To Default"() -> ()  [unwired: 3 in, 3 out]
            n160 = invoke on="Frame #" class="DigNum (strict)" method="Reinit To Default"() -> ()  [unwired: 3 in, 3 out]
            n161 = invoke on="Det 6" class="DigNum (strict)" method="Reinit To Default"() -> ()  [unwired: 3 in, 3 out]
            n162 = invoke on="Det 2" class="DigNum (strict)" method="Reinit To Default"() -> ()  [unwired: 3 in, 3 out]
            n163 = invoke on="Det 1" class="DigNum (strict)" method="Reinit To Default"() -> ()  [unwired: 3 in, 3 out]
            n164 = invoke on="g2" class="XYGraph (strict)" method="Reinit To Default"() -> ()  [unwired: 3 in, 3 out]
            n165 = invoke on="Trial #" class="DigNum (strict)" method="Reinit To Default"() -> ()  [unwired: 3 in, 3 out]
            n166 = property on="Tau" class="WFChart (strict)"("History Data"=cluster{"tmp":dbl, dbl}[] []) -> ()  [unwired: 2 in, 2 out]
            n167 = case shown="\"8 Detectors\", Default" w176 {
              tunnel: [w180 w182] -> w178
              tunnel: [TRUE FALSE] -> w175
              frame "4 Detectors" {
                n168 = dll-call lib="C:/Users/BUCKLEY-ADMIN/Desktop/DCScode_simulISS_MAP/flex05-4chPascal.dll" fn="USBInitialize" label="InitCH4"() -> ("return type"=w180:u8)  [unwired: 3 in, 2 out]
              }
              frame "8 Detectors", Default {
                n169 = dll-call lib="C:/Users/BUCKLEY-ADMIN/Desktop/DCScode_simulISS_MAP/flex05oem8chauto100nsPASCAL_win7.dll" fn="USBInitialize" label="InitCH8"() -> ("return type"=w182:u8)  [unwired: 3 in, 2 out]
              }
            }
            "4CH?" <- w175
            n170 = Equal To 0?(x=w178) -> (x = 0?=w177:bool)
            n171 = call "Display Message to User2"("Enable"=w177, "Message"="ATTENTION:\nPROBLEM WITH CORRELATOR!") -> ()  [unwired: 8 in, 2 out]
          }
          event "Sequence Scan": Value Change {
            # "Initialize Baseline"
            n172 = event-data() -> ()  [unwired: 1 in, 6 out]
            n173 = case shown="\"8 Detectors\", Default" w185 {
              tunnel: [w668 w669] -> w186
              frame "4 Detectors" {
                n174 = local read "4CH?"() -> (w668:bool)
              }
              frame "8 Detectors", Default {
                # "Select whether using\n 4 or 8ch correlator"
                n175 = local read "4CH?"() -> (w670:bool)
                n176 = Not(x=w670) -> (.not. x?=w669:bool)
              }
            }
            n177 = case shown="True" w186 {
              selector: w186 -> [w191 _]
              tunnel: w184 -> [_ w205]
              tunnel: w185 -> [_ w206]
              tunnel: sgl 1.0 -> [_ w193]
              frame False {
                n178 = invoke on="Sequence Scan" class="Bool" method="Reinit To Default"() -> ()  [unwired: 3 in, 3 out]
                n179 = Not(x=w191) -> (.not. x?=w190:bool)
                n180 = call "Display Message to User3"("Enable"=w190, "Message"="ATTENTION:\nYou have changed Detector Select,\nplease press Initialize Correlator first!") -> ()  [unwired: 8 in, 2 out]
              }
              frame True {
                # "This part pauses and alerts user that test function is on. If test function is accepted then code runs but data is not saved (no timestamp either)."
                # "This checks for if the file already exists in the directory using the timing file. \n*If YES, then we don't do anything to the lasers. We just display message and wait for the user to input a new name and press sequence again.\n*If NO, then we proceed as per normal."
                n181 = case shown="True" "Test" {
                  selector: "Test" -> [w208 _]
                  tunnel: "Test" -> [_ w210]
                  tunnel: [w207 w209] -> w194
                  frame False {
                    n182 = Not(x=w208) -> (.not. x?=w207:bool)
                  }
                  frame True {
                    n183 = call "Test ON"("Enable"=w210) -> ("No - STOP"=w211:bool, "OK"=w209:bool)  [unwired: 15 in, 2 out]
                    n184 = local write "Stop"(w211) -> ()
                  }
                }
                n185 = local read "File Name:"() -> (w201:string)
                n186 = local read "Data Save Directory:"() -> (w200:path)
                n187 = Concatenate Strings(w201, "_TIMING", ".dat") -> (w203:string)
                n188 = Build Path(base path=w200, name or relative path=w203) -> (appended path=w199:path)
                n189 = call <vilib>:"Check if File or Folder Exists.vi"("path"=w199) -> ("file or folder exists?"=w196:bool)  [unwired: 8 in, 2 out]
                n190 = Not(x=w196) -> (.not. x?=w198:bool)
                n191 = Not And(1:w194, 2:w198) -> (0:w197:bool)
                n192 = case shown="False" w197 {
                  tunnel: w206 -> [w213 _]
                  tunnel: w205 -> [w214 _]
                  tunnel: w193 -> [w215 _]
                  frame False {
                    # "Turn relay on so that Optical switch is open and LED indicator is ON"
                    # "When the START button is pressed, the ISS lasers turn off"
                    n193 = local read "Fixed # of Frames"() -> (w220:u32)
                    n194 = Build Array(TRUE, TRUE) -> (w225:bool[])
                    n195 = call "DAQ Assistant"("data"=w225) -> ()  [unwired: 17 in, 2 out]
                    n196 = Initialize Array "Initialize Array"(nan, w220) -> (w212:dbl[])
                    n197 = while {
                      tunnel: w213 -> [w239]
                      tunnel: w214 -> [w269]
                      tunnel: w215 -> [_]
                      shift-right: [w242] -> _
                      shift-left: w212 -> [w243]
                      stop <- w244 stop-if-true
                      # "Only runs Real Time Fitting if \nReal Time Fitting box is checked \nand test function is off."
                      # "After testing is complete, turn off the lasers and\nreset  the buttons."
                      n198 = Index Array(array="Visible\nAverages", index=3) -> (element=w262:bool)
                      n199 = Index Array(array="Visible\nAverages", index=1) -> (element=w263:bool)
                      n200 = Index Array(array="Visible\nAverages", index=0) -> (element=w256:bool)
                      n201 = Index Array(array="Visible\nAverages", index=2) -> (element=w257:bool)
                      n202 = property on="Tau 2" class="WFChart (strict)"("Active Plot"=u32 11) -> (error out=w260:errorcluster)  [unwired: 2 in, 1 out]
                      n203 = property on="Tau 2" class="WFChart (strict)"("Active Plot"=u32 9) -> (error out=w265:errorcluster)  [unwired: 2 in, 1 out]
                      n204 = property on="Tau 2" class="WFChart (strict)"("Active Plot"=u32 8) -> (error out=w254:errorcluster)  [unwired: 2 in, 1 out]
                      n205 = property on="Tau 2" class="WFChart (strict)"("Active Plot"=u32 10) -> (error out=w259:errorcluster)  [unwired: 2 in, 1 out]
                      n206 = property on="Tau 2" class="WFChart (strict)"(error in=w260, "Plot.Visible?"=w262) -> ()  [unwired: 1 in, 2 out]
                      n207 = property on="Tau 2" class="WFChart (strict)"(error in=w265, "Plot.Visible?"=w263) -> ()  [unwired: 1 in, 2 out]
                      n208 = property on="Tau 2" class="WFChart (strict)"(error in=w254, "Plot.Visible?"=w256) -> ()  [unwired: 1 in, 2 out]
                      n209 = property on="Tau 2" class="WFChart (strict)"(error in=w259, "Plot.Visible?"=w257) -> ()  [unwired: 1 in, 2 out]
                      n210 = for {
                        N: 1 -> [_]
                        tunnel: w269 -> [w310]
                        tunnel: w239 -> [w309]
                        tunnel: [w306] -> w244
                        tunnel: [w305] -> w268
                        tunnel: [w303] -> w248
                        tunnel: [w301] -> w247
                        tunnel: [w302] -> w246
                        # "The logic here may look funny but it works elegantly. No matter if you choose \"Use Both Lasers\", the AND output is always\nfalse the first time these two boxes run since Laser 1 Value is always false, and the default is to use flow laser 1.\nBUT, the trick is if you chose \"Use Both Laser\" This big for loop is gonna run twice, the second time it runs, \nthe laser 1 value is TRUE because it is set to TRUE by the second box when the big for loop ran the first time. Now, when\nthe output of AND is true, ISS laser no longer runs. Only flow laser two is turned on and we execute the for loop to the right."
                        # "These two boxes take care of the flow chart.\nIt turn on ISS laser first, then triggers it and turn it off.\nIf ISS data is ready, then we go on to flow lase."
                        # "This loop may seem useless but it acts as a block. \nThis block does all the data collection, plotting and writing the data\nto file"
                        n211 = case shown="\"8 Detectors\", Default" w309 {
                          selector: w309 -> [w666 w667]
                          tunnel: [w666 w667] -> w307
                          frame "4 Detectors" {
                            n212 = dll-call lib="C:/Users/BUCKLEY-ADMIN/Desktop/DCScode_simulISS_MAP/flex05-4chPascal.dll" fn="USBStart" label="StartCH4"() -> ()  [unwired: 4 in, 2 out]
                          }
                          frame "8 Detectors", Default {
                            n213 = dll-call lib="C:/Users/BUCKLEY-ADMIN/Desktop/DCScode_simulISS_MAP/flex05oem8chauto100nsPASCAL_win7.dll" fn="USBStart" label="StartCH8"() -> ()  [unwired: 4 in, 2 out]
                          }
                        }
                        n214 = for {
                          N: 1 -> [_]
                          tunnel: w310 -> [w334]
                          tunnel: [w314] -> w306
                          tunnel: w307 -> [w311]
                          tunnel: [w316] -> w305
                          tunnel: "MARK\nMark" -> [w328]
                          tunnel: [w315] -> w303
                          tunnel: [w313] -> w301
                          tunnel: [w327] -> w302
                          w320 = FALSE
                          w312 = u8 2
                          # "Only saves data if\ntest function is off."
                          # "If Fixed # Frames check box is selected,\ncode will run for # of frames specified on \nfront panel and then call Stop button"
                          # "This for loop here acts as a block as well. It takes the relative \nflow data from UpdateData.vi and plot the data on the graph.\nWhen \"Baseline\" is selected,  the data point goes to 1. When\n\"Mark\" is selected, a point at positive infinity is plotted and a\nvertical line joining the point and the x axis if displayed."
                          n215 = Current VI's Menubar() -> (w336:refnum<k9>)
                          n216 = Set Menu Item Info(7:"File", 9:w320, 11:w336) -> (3:w335:refnum<k9>)  [unwired: 4 in, 1 out]
                          n217 = Set Menu Item Info(7:"Options", 9:w320, 11:w335) -> ()  [unwired: 4 in, 2 out]
                          n218 = while {
                            tunnel: [w522] -> w342
                            tunnel: [w492] -> w341
                            tunnel: [w493] -> w340
                            tunnel: [w496] -> w314
                            tunnel: [w523] -> w339
                            tunnel: w334 -> [w525]
                            tunnel: w311 -> [w498]
                            stop <- w527 stop-if-true
                            # "D4 Tail Alarm"
                            # "D2 Tail Alarm"
                            # "D8 Tail Alarm"
                            # "D7 Tail Alarm"
                            # "D6 Tail Alarm"
                            # "D5 Tail Alarm"
                            # "D3 Tail Alarm"
                            # "D1 Tail Alarm"
                            # "When press STOP, turn off DCS laser LED indicator is OFF"
                            n219 = Not(x="D4") -> (.not. x?=w511:bool)
                            n220 = Not(x="D8") -> (.not. x?=w507:bool)
                            n221 = Not(x="D5") -> (.not. x?=w510:bool)
                            n222 = Not(x="D1") -> (.not. x?=w514:bool)
                            n223 = Not(x="D6") -> (.not. x?=w509:bool)
                            n224 = Not(x="D2") -> (.not. x?=w499:bool)
                            n225 = Not(x="D7") -> (.not. x?=w508:bool)
                            n226 = Not(x="D3") -> (.not. x?=w512:bool)
                            n227 = case shown="True" "Stop" {
                              selector: "Stop" -> [w566 w572]
                              tunnel: [w566 w569] -> w496
                              frame False {
                              }
                              frame True {
                                n228 = call "Prompt User for Input"("Enable"=w572) -> ("Yes"=w569:bool)  [unwired: 17 in, 1 out]
                                n229 = Build Array(w569, FALSE) -> (w571:bool[])
                                n230 = call "DAQ Assistant2"("data"=w571) -> ()  [unwired: 17 in, 2 out]
                                n231 = local read "Laser Input Name"() -> (w567:refnum<visa-resource-name>)
                                n232 = call "iBs.vi"("Laser On/Off"=FALSE, "VISA resource name"=w567) -> ()
                              }
                            }
                            n233 = case shown="True" "Clear plots" {
                              frame False {
                              }
                              frame True {
                                n234 = invoke on="g2" class="XYGraph (strict)" method="Reinit To Default"() -> ()  [unwired: 3 in, 3 out]
                              }
                            }
                            n235 = case shown="False" w511 {
                              selector: w511 -> [w613 w618]
                              frame False {
                                n236 = property on="Tau 2" class="WFChart (strict)"("Active Plot"=u32 3) -> (error out=w615:errorcluster)  [unwired: 2 in, 1 out]
                                n237 = property on="g2" class="XYGraph (strict)"("Active Plot"=u32 3) -> (error out=w616:errorcluster)  [unwired: 2 in, 1 out]
                                n238 = property on="g2" class="XYGraph (strict)"(error in=w616, "Plot.Visible?"=w613) -> ()  [unwired: 1 in, 2 out]
                                n239 = property on="Tau 2" class="WFChart (strict)"(error in=w615, "Plot.Visible?"=w613) -> ()  [unwired: 1 in, 2 out]
                              }
                              frame True {
                                n240 = property on="Tau 2" class="WFChart (strict)"("Active Plot"=u32 3) -> (error out=w619:errorcluster)  [unwired: 2 in, 1 out]
                                n241 = property on="Tau 2" class="WFChart (strict)"(error in=w619, "Plot.Visible?"=w618) -> ()  [unwired: 1 in, 2 out]
                                n242 = property on="g2" class="XYGraph (strict)"("Active Plot"=u32 3) -> (error out=w621:errorcluster)  [unwired: 2 in, 1 out]
                                n243 = property on="g2" class="XYGraph (strict)"(error in=w621, "Plot.Visible?"=w618) -> ()  [unwired: 1 in, 2 out]
                              }
                            }
                            n244 = case shown="False" w507 {
                              selector: w507 -> [w573 w578]
                              frame False {
                                n245 = property on="Tau 2" class="WFChart (strict)"("Active Plot"=u32 7) -> (error out=w574:errorcluster)  [unwired: 2 in, 1 out]
                                n246 = property on="g2" class="XYGraph (strict)"("Active Plot"=u32 7) -> (error out=w576:errorcluster)  [unwired: 2 in, 1 out]
                                n247 = property on="g2" class="XYGraph (strict)"(error in=w576, "Plot.Visible?"=w573) -> ()  [unwired: 1 in, 2 out]
                                n248 = property on="Tau 2" class="WFChart (strict)"(error in=w574, "Plot.Visible?"=w573) -> ()  [unwired: 1 in, 2 out]
                              }
                              frame True {
                                n249 = property on="Tau 2" class="WFChart (strict)"("Active Plot"=u32 7) -> (error out=w580:errorcluster)  [unwired: 2 in, 1 out]
                                n250 = property on="Tau 2" class="WFChart (strict)"(error in=w580, "Plot.Visible?"=w578) -> ()  [unwired: 1 in, 2 out]
                                n251 = property on="g2" class="XYGraph (strict)"("Active Plot"=u32 7) -> (error out=w581:errorcluster)  [unwired: 2 in, 1 out]
                                n252 = property on="g2" class="XYGraph (strict)"(error in=w581, "Plot.Visible?"=w578) -> ()  [unwired: 1 in, 2 out]
                              }
                            }
                            n253 = case shown="False" w510 {
                              selector: w510 -> [w603 w608]
                              frame False {
                                n254 = property on="Tau 2" class="WFChart (strict)"("Active Plot"=u32 4) -> (error out=w605:errorcluster)  [unwired: 2 in, 1 out]
                                n255 = property on="g2" class="XYGraph (strict)"("Active Plot"=u32 4) -> (error out=w606:errorcluster)  [unwired: 2 in, 1 out]
                                n256 = property on="g2" class="XYGraph (strict)"(error in=w606, "Plot.Visible?"=w603) -> ()  [unwired: 1 in, 2 out]
                                n257 = property on="Tau 2" class="WFChart (strict)"(error in=w605, "Plot.Visible?"=w603) -> ()  [unwired: 1 in, 2 out]
                              }
                              frame True {
                                n258 = property on="Tau 2" class="WFChart (strict)"("Active Plot"=u32 4) -> (error out=w610:errorcluster)  [unwired: 2 in, 1 out]
                                n259 = property on="Tau 2" class="WFChart (strict)"(error in=w610, "Plot.Visible?"=w608) -> ()  [unwired: 1 in, 2 out]
                                n260 = property on="g2" class="XYGraph (strict)"("Active Plot"=u32 4) -> (error out=w611:errorcluster)  [unwired: 2 in, 1 out]
                                n261 = property on="g2" class="XYGraph (strict)"(error in=w611, "Plot.Visible?"=w608) -> ()  [unwired: 1 in, 2 out]
                              }
                            }
                            n262 = case shown="False" w514 {
                              selector: w514 -> [w643 w648]
                              frame False {
                                n263 = property on="Tau 2" class="WFChart (strict)"("Active Plot"=u32 0) -> (error out=w644:errorcluster)  [unwired: 2 in, 1 out]
                                n264 = property on="g2" class="XYGraph (strict)"("Active Plot"=u32 0) -> (error out=w646:errorcluster)  [unwired: 2 in, 1 out]
                                n265 = property on="g2" class="XYGraph (strict)"(error in=w646, "Plot.Visible?"=w643) -> ()  [unwired: 1 in, 2 out]
                                n266 = property on="Tau 2" class="WFChart (strict)"(error in=w644, "Plot.Visible?"=w643) -> ()  [unwired: 1 in, 2 out]
                              }
                              frame True {
                                n267 = property on="Tau 2" class="WFChart (strict)"("Active Plot"=u32 0) -> (error out=w650:errorcluster)  [unwired: 2 in, 1 out]
                                n268 = property on="Tau 2" class="WFChart (strict)"(error in=w650, "Plot.Visible?"=w648) -> ()  [unwired: 1 in, 2 out]
                                n269 = property on="g2" class="XYGraph (strict)"("Active Plot"=u32 0) -> (error out=w651:errorcluster)  [unwired: 2 in, 1 out]
                                n270 = property on="g2" class="XYGraph (strict)"(error in=w651, "Plot.Visible?"=w648) -> ()  [unwired: 1 in, 2 out]
                              }
                            }
                            n271 = case shown="False" w509 {
                              selector: w509 -> [w593 w598]
                              frame False {
                                n272 = property on="Tau 2" class="WFChart (strict)"("Active Plot"=u32 5) -> (error out=w595:errorcluster)  [unwired: 2 in, 1 out]
                                n273 = property on="g2" class="XYGraph (strict)"("Active Plot"=u32 5) -> (error out=w596:errorcluster)  [unwired: 2 in, 1 out]
                                n274 = property on="g2" class="XYGraph (strict)"(error in=w596, "Plot.Visible?"=w593) -> ()  [unwired: 1 in, 2 out]
                                n275 = property on="Tau 2" class="WFChart (strict)"(error in=w595, "Plot.Visible?"=w593) -> ()  [unwired: 1 in, 2 out]
                              }
                              frame True {
                                n276 = property on="Tau 2" class="WFChart (strict)"("Active Plot"=u32 5) -> (error out=w599:errorcluster)  [unwired: 2 in, 1 out]
                                n277 = property on="Tau 2" class="WFChart (strict)"(error in=w599, "Plot.Visible?"=w598) -> ()  [unwired: 1 in, 2 out]
                                n278 = property on="g2" class="XYGraph (strict)"("Active Plot"=u32 5) -> (error out=w601:errorcluster)  [unwired: 2 in, 1 out]
                                n279 = property on="g2" class="XYGraph (strict)"(error in=w601, "Plot.Visible?"=w598) -> ()  [unwired: 1 in, 2 out]
                              }
                            }
                            n280 = case shown="False" w499 {
                              selector: w499 -> [w633 w638]
                              frame False {
                                n281 = property on="Tau 2" class="WFChart (strict)"("Active Plot"=u32 1) -> (error out=w635:errorcluster)  [unwired: 2 in, 1 out]
                                n282 = property on="g2" class="XYGraph (strict)"("Active Plot"=u32 1) -> (error out=w636:errorcluster)  [unwired: 2 in, 1 out]
                                n283 = property on="g2" class="XYGraph (strict)"(error in=w636, "Plot.Visible?"=w633) -> ()  [unwired: 1 in, 2 out]
                                n284 = property on="Tau 2" class="WFChart (strict)"(error in=w635, "Plot.Visible?"=w633) -> ()  [unwired: 1 in, 2 out]
                              }
                              frame True {
                                n285 = property on="Tau 2" class="WFChart (strict)"("Active Plot"=u32 1) -> (error out=w640:errorcluster)  [unwired: 2 in, 1 out]
                                n286 = property on="Tau 2" class="WFChart (strict)"(error in=w640, "Plot.Visible?"=w638) -> ()  [unwired: 1 in, 2 out]
                                n287 = property on="g2" class="XYGraph (strict)"("Active Plot"=u32 1) -> (error out=w641:errorcluster)  [unwired: 2 in, 1 out]
                                n288 = property on="g2" class="XYGraph (strict)"(error in=w641, "Plot.Visible?"=w638) -> ()  [unwired: 1 in, 2 out]
                              }
                            }
                            n289 = case shown="False" w508 {
                              selector: w508 -> [w583 w588]
                              frame False {
                                n290 = property on="Tau 2" class="WFChart (strict)"("Active Plot"=u32 6) -> (error out=w585:errorcluster)  [unwired: 2 in, 1 out]
                                n291 = property on="g2" class="XYGraph (strict)"("Active Plot"=u32 6) -> (error out=w586:errorcluster)  [unwired: 2 in, 1 out]
                                n292 = property on="g2" class="XYGraph (strict)"(error in=w586, "Plot.Visible?"=w583) -> ()  [unwired: 1 in, 2 out]
                                n293 = property on="Tau 2" class="WFChart (strict)"(error in=w585, "Plot.Visible?"=w583) -> ()  [unwired: 1 in, 2 out]
                              }
                              frame True {
                                n294 = property on="Tau 2" class="WFChart (strict)"("Active Plot"=u32 6) -> (error out=w589:errorcluster)  [unwired: 2 in, 1 out]
                                n295 = property on="Tau 2" class="WFChart (strict)"(error in=w589, "Plot.Visible?"=w588) -> ()  [unwired: 1 in, 2 out]
                                n296 = property on="g2" class="XYGraph (strict)"("Active Plot"=u32 6) -> (error out=w591:errorcluster)  [unwired: 2 in, 1 out]
                                n297 = property on="g2" class="XYGraph (strict)"(error in=w591, "Plot.Visible?"=w588) -> ()  [unwired: 1 in, 2 out]
                              }
                            }
                            n298 = case shown="False" w512 {
                              selector: w512 -> [w623 w628]
                              frame False {
                                n299 = property on="Tau 2" class="WFChart (strict)"("Active Plot"=u32 2) -> (error out=w624:errorcluster)  [unwired: 2 in, 1 out]
                                n300 = property on="g2" class="XYGraph (strict)"("Active Plot"=u32 2) -> (error out=w626:errorcluster)  [unwired: 2 in, 1 out]
                                n301 = property on="g2" class="XYGraph (strict)"(error in=w626, "Plot.Visible?"=w623) -> ()  [unwired: 1 in, 2 out]
                                n302 = property on="Tau 2" class="WFChart (strict)"(error in=w624, "Plot.Visible?"=w623) -> ()  [unwired: 1 in, 2 out]
                              }
                              frame True {
                                n303 = property on="Tau 2" class="WFChart (strict)"("Active Plot"=u32 2) -> (error out=w630:errorcluster)  [unwired: 2 in, 1 out]
                                n304 = property on="Tau 2" class="WFChart (strict)"(error in=w630, "Plot.Visible?"=w628) -> ()  [unwired: 1 in, 2 out]
                                n305 = property on="g2" class="XYGraph (strict)"("Active Plot"=u32 2) -> (error out=w631:errorcluster)  [unwired: 2 in, 1 out]
                                n306 = property on="g2" class="XYGraph (strict)"(error in=w631, "Plot.Visible?"=w628) -> ()  [unwired: 1 in, 2 out]
                              }
                            }
                            n307 = Wait (ms)(milliseconds to wait="Update Time (ms)\nDO NOT CHANGE!") -> ()  [unwired: 1 out]
                            n308 = call "UpdateData.vi"("Duration Time (ms)"="Integration Time (ms)", "Detector Select"=w498, "Delay Time"=w525) -> ("Elapsed Time(s)"=w526:sgl, "Intensity Array"=w524:sgl[], "Tau Array"=w523:sgl[], "mean"=w488:dbl, "mean 8"=w468:dbl, "mean 2"=w437:dbl, "mean 7"=w469:dbl, "mean 3"=w473:dbl, "Intensity data"=w522:string, "g2 Display"=→"g2":cluster{"Delay Time":sgl[], sgl[]}[], "mean 4"=w472:dbl, "mean 5"=w471:dbl, "mean 6"=w470:dbl, "tau data"=w492:string, "g2 data"=w493:string)  [unwired: 2 in]
                            n309 = Multiply(x=sgl 1000.0, y=w526) -> (x*y=w530:sgl)
                            n310 = Less?(x=w488, y=1.005) -> (x < y?=w467:bool)
                            n311 = Less?(x=w437, y=1.005) -> (x < y?=w421:bool)
                            n312 = Less?(x=w473, y=1.005) -> (x < y?=w420:bool)
                            n313 = Less?(x=w472, y=1.005) -> (x < y?=w417:bool)
                            n314 = Less?(x=w471, y=1.005) -> (x < y?=w415:bool)
                            n315 = Less?(x=w470, y=1.005) -> (x < y?=w413:bool)
                            n316 = Less?(x=w469, y=1.005) -> (x < y?=w411:bool)
                            n317 = Less?(x=w468, y=1.005) -> (x < y?=w409:bool)
                            n318 = Index Array(array=w524, index #1=0, index #2=1, index #3=2, index #4=3, index #5=4, index #6=5, index #7=6, index #8=7) -> (element #1=w465:sgl, element #2=w444:sgl, element #3=w443:sgl, element #4=w442:sgl, element #5=w441:sgl, element #6=w440:sgl, element #7=w439:sgl, element #8=w438:sgl)
                            "Det 7" <- w439
                            "Det 6" <- w440
                            "Det 5" <- w441
                            "Det 4" <- w442
                            "Det 3" <- w443
                            "Det 2" <- w444
                            "Det 1" <- w465
                            "Det 8" <- w438
                            n319 = Subtract(x="Integration Time (ms)", y=w530) -> (x-y=w528:sgl)
                            "Time Left (ms)" <- w528
                            n320 = Greater?(x=w488, y=0.98) -> (0:w466:bool)
                            n321 = Greater?(x=w472, y=0.98) -> (0:w418:bool)
                            n322 = Greater?(x=w470, y=0.98) -> (0:w414:bool)
                            n323 = Greater?(x=w468, y=0.98) -> (0:w410:bool)
                            n324 = Greater Or Equal?(x=w465, y=sgl 2.0) -> (x >= y?=w462:bool)
                            n325 = Greater Or Equal?(x=w444, y=sgl 2.0) -> (x >= y?=w408:bool)
                            n326 = Greater Or Equal?(x=w443, y=sgl 2.0) -> (x >= y?=w406:bool)
                            n327 = Greater Or Equal?(x=w442, y=sgl 2.0) -> (x >= y?=w404:bool)
                            n328 = Greater Or Equal?(x=w441, y=sgl 2.0) -> (x >= y?=w402:bool)
                            n329 = Greater Or Equal?(x=w440, y=sgl 2.0) -> (x >= y?=w400:bool)
                            n330 = Less Or Equal?(x=w465, y=sgl 1000.0) -> (x <= y?=w461:bool)
                            n331 = Less Or Equal?(x=w444, y=sgl 1000.0) -> (x <= y?=w407:bool)
                            n332 = Less Or Equal?(x=w443, y=sgl 1000.0) -> (x <= y?=w405:bool)
                            n333 = Less Or Equal?(x=w442, y=sgl 1000.0) -> (x <= y?=w403:bool)
                            n334 = Less Or Equal?(x=w441, y=sgl 1000.0) -> (x <= y?=w401:bool)
                            n335 = Less Or Equal?(x=w440, y=sgl 1000.0) -> (x <= y?=w399:bool)
                            n336 = Less Or Equal?(x=w439, y=sgl 1000.0) -> (x <= y?=w397:bool)
                            n337 = Less Or Equal?(x=w438, y=sgl 1000.0) -> (x <= y?=w395:bool)
                            n338 = Greater Or Equal?(x=w439, y=sgl 2.0) -> (x >= y?=w398:bool)
                            n339 = Greater Or Equal?(x=w438, y=sgl 2.0) -> (x >= y?=w396:bool)
                            n340 = Greater?(x=w437, y=0.98) -> (0:w422:bool)
                            n341 = Greater?(x=w473, y=0.98) -> (0:w419:bool)
                            n342 = Greater?(x=w471, y=0.98) -> (0:w416:bool)
                            n343 = Greater?(x=w469, y=0.98) -> (0:w412:bool)
                            n344 = Build Array(w467, w466, w462, w461) -> (w460:bool[])
                            n345 = Build Array(w422, w421, w408, w407) -> (w436:bool[])
                            n346 = Build Array(w420, w419, w406, w405) -> (w435:bool[])
                            n347 = Build Array(w418, w417, w404, w403) -> (w434:bool[])
                            n348 = Build Array(w416, w415, w402, w401) -> (w433:bool[])
                            n349 = Build Array(w414, w413, w400, w399) -> (w432:bool[])
                            n350 = Build Array(w412, w411, w398, w397) -> (w431:bool[])
                            n351 = Build Array(w410, w409, w396, w395) -> (w430:bool[])
                            n352 = And Array Elements(Boolean array=w460) -> (logical AND=w459:bool)
                            n353 = And Array Elements(Boolean array=w436) -> (logical AND=w423:bool)
                            n354 = And Array Elements(Boolean array=w435) -> (logical AND=w424:bool)
                            n355 = And Array Elements(Boolean array=w434) -> (logical AND=w425:bool)
                            n356 = And Array Elements(Boolean array=w433) -> (logical AND=w426:bool)
                            n357 = And Array Elements(Boolean array=w432) -> (logical AND=w427:bool)
                            n358 = And Array Elements(Boolean array=w431) -> (logical AND=w428:bool)
                            n359 = And Array Elements(Boolean array=w430) -> (logical AND=w429:bool)
                            n360 = Less Or Equal To 0?(x=w528) -> (x <= 0?=w529:bool)
                            n361 = case shown="True" w459 {
                              frame False {
                                n362 = control-ref of="Det 1"() -> (w562:refnum<vi>)
                                n363 = property on="Property Node" class="Digital (strict)"(reference=w562, "DisabledEnum"=T5."Disabled and Grayed Out" ("Disabled")) -> ()  [unwired: 1 in, 2 out]
                              }
                              frame True {
                                n364 = control-ref of="Det 1"() -> (w564:refnum<vi>)
                                n365 = property on="Property Node" class="Digital (strict)"(reference=w564, "DisabledEnum"=T5."Enabled" ("Disabled")) -> ()  [unwired: 1 in, 2 out]
                              }
                            }
                            n366 = case shown="True" w423 {
                              frame False {
                                n367 = control-ref of="Det 2"() -> (w558:refnum<vi>)
                                n368 = property on="Property Node" class="Digital (strict)"(reference=w558, "DisabledEnum"=T5."Disabled and Grayed Out" ("Disabled")) -> ()  [unwired: 1 in, 2 out]
                              }
                              frame True {
                                n369 = control-ref of="Det 2"() -> (w560:refnum<vi>)
                                n370 = property on="Property Node" class="Digital (strict)"(reference=w560, "DisabledEnum"=T5."Enabled" ("Disabled")) -> ()  [unwired: 1 in, 2 out]
                              }
                            }
                            n371 = case shown="True" w424 {
                              frame False {
                                n372 = control-ref of="Det 3"() -> (w554:refnum<vi>)
                                n373 = property on="Property Node" class="Digital (strict)"(reference=w554, "DisabledEnum"=T5."Disabled and Grayed Out" ("Disabled")) -> ()  [unwired: 1 in, 2 out]
                              }
                              frame True {
                                n374 = control-ref of="Det 3"() -> (w556:refnum<vi>)
                                n375 = property on="Property Node" class="Digital (strict)"(reference=w556, "DisabledEnum"=T5."Enabled" ("Disabled")) -> ()  [unwired: 1 in, 2 out]
                              }
                            }
                            n376 = case shown="True" w425 {
                              frame False {
                                n377 = control-ref of="Det 4"() -> (w550:refnum<vi>)
                                n378 = property on="Property Node" class="Digital (strict)"(reference=w550, "DisabledEnum"=T5."Disabled and Grayed Out" ("Disabled")) -> ()  [unwired: 1 in, 2 out]
                              }
                              frame True {
                                n379 = control-ref of="Det 4"() -> (w552:refnum<vi>)
                                n380 = property on="Property Node" class="Digital (strict)"(reference=w552, "DisabledEnum"=T5."Enabled" ("Disabled")) -> ()  [unwired: 1 in, 2 out]
                              }
                            }
                            n381 = case shown="True" w426 {
                              frame False {
                                n382 = control-ref of="Det 5"() -> (w546:refnum<vi>)
                                n383 = property on="Property Node" class="Digital (strict)"(reference=w546, "DisabledEnum"=T5."Disabled and Grayed Out" ("Disabled")) -> ()  [unwired: 1 in, 2 out]
                              }
                              frame True {
                                n384 = control-ref of="Det 5"() -> (w548:refnum<vi>)
                                n385 = property on="Property Node" class="Digital (strict)"(reference=w548, "DisabledEnum"=T5."Enabled" ("Disabled")) -> ()  [unwired: 1 in, 2 out]
                              }
                            }
                            n386 = case shown="False" w427 {
                              frame False {
                                n387 = control-ref of="Det 6"() -> (w542:refnum<vi>)
                                n388 = property on="Property Node" class="Digital (strict)"(reference=w542, "DisabledEnum"=T5."Disabled and Grayed Out" ("Disabled")) -> ()  [unwired: 1 in, 2 out]
                              }
                              frame True {
                                n389 = control-ref of="Det 6"() -> (w544:refnum<vi>)
                                n390 = property on="Property Node" class="Digital (strict)"(reference=w544, "DisabledEnum"=T5."Enabled" ("Disabled")) -> ()  [unwired: 1 in, 2 out]
                              }
                            }
                            n391 = case shown="True" w428 {
                              frame False {
                                n392 = control-ref of="Det 7"() -> (w538:refnum<vi>)
                                n393 = property on="Property Node" class="Digital (strict)"(reference=w538, "DisabledEnum"=T5."Disabled and Grayed Out" ("Disabled")) -> ()  [unwired: 1 in, 2 out]
                              }
                              frame True {
                                n394 = control-ref of="Det 7"() -> (w540:refnum<vi>)
                                n395 = property on="Property Node" class="Digital (strict)"(reference=w540, "DisabledEnum"=T5."Enabled" ("Disabled")) -> ()  [unwired: 1 in, 2 out]
                              }
                            }
                            n396 = case shown="True" w429 {
                              frame False {
                                n397 = control-ref of="Det 8"() -> (w534:refnum<vi>)
                                n398 = property on="Property Node" class="Digital (strict)"(reference=w534, "DisabledEnum"=T5."Disabled and Grayed Out" ("Disabled")) -> ()  [unwired: 1 in, 2 out]
                              }
                              frame True {
                                n399 = control-ref of="Det 8"() -> (w536:refnum<vi>)
                                n400 = property on="Property Node" class="Digital (strict)"(reference=w536, "DisabledEnum"=T5."Enabled" ("Disabled")) -> ()  [unwired: 1 in, 2 out]
                              }
                            }
                            n401 = Or(x=w496, y=w529) -> (x .or. y?=w527:bool)
                            n402 = case shown="True" w527 {
                              tunnel: w498 -> [w653 _]
                              frame True {
                                n403 = case shown="\"8 Detectors\", Default" w653 {
                                frame "4 Detectors" {
                                n404 = dll-call lib="C:/Users/BUCKLEY-ADMIN/Desktop/DCScode_simulISS_MAP/flex05-4chPascal.dll" fn="USBStop" label="StopCH4"() -> ()  [unwired: 4 in, 2 out]
                                }
                                frame "8 Detectors", Default {
                                n405 = dll-call lib="C:/Users/BUCKLEY-ADMIN/Desktop/DCScode_simulISS_MAP/flex05oem8chauto100nsPASCAL_win7.dll" fn="USBStop" label="StopCH8"() -> ()  [unwired: 4 in, 2 out]
                                }
                                }
                              }
                              frame False {
                              }
                            }
                          }
                          n406 = local read "Trial #"() -> (w331:u32)
                          n407 = property on="QUIT" class="Bool (strict)"("Disabled"=w312) -> ()  [unwired: 2 in, 2 out]
                          n408 = Increment(x=w331) -> (x+1=w330:u32)
                          n409 = property on="Sequence Scan" class="Bool"("Disabled"=w312) -> ()  [unwired: 2 in, 2 out]
                          n410 = local write "Trial #"(w330) -> ()
                          n411 = property on="Update Time (ms)\nDO NOT CHANGE!" class="DigNum (strict)"("Disabled"=w312) -> ()  [unwired: 2 in, 2 out]
                          n412 = property on="Integration Time (ms)" class="DigNum (strict)"("Disabled"=w312) -> ()  [unwired: 2 in, 2 out]
                          n413 = property on="Detector Select" class="RadioBtnsControl (strict)"("Disabled"=w312) -> ()  [unwired: 2 in, 2 out]
                          n414 = property on="Initialize Correlator" class="Bool"("Disabled"=w312) -> ()  [unwired: 2 in, 2 out]
                          n415 = case shown="\"Det 2\"" "Detector Used" {
                            tunnel: [1 2 3 4 5 6 7 8] -> w333
                            frame "Det 1", Default {
                            }
                            frame "Det 2" {
                            }
                            frame "Det 3" {
                            }
                            frame "Det 4" {
                            }
                            frame "Det 5" {
                            }
                            frame "Det 6" {
                            }
                            frame "Det 7" {
                            }
                            frame "Det 8" {
                            }
                          }
                          n416 = for {
                            N: 1 -> [_]
                            tunnel: w339 -> [w383]
                            tunnel: [w386] -> w319
                            tunnel: w333 -> [w385]
                            tunnel: w328 -> [w376]
                            n417 = Index Array(array=w383, index=w385) -> (element=w384:sgl)
                            n418 = Boolean To (0,1)(Boolean="Baseline") -> (0, 1=w388:i16)
                            n419 = case shown="True" w376 {
                              tunnel: [0.0 w390] -> w380
                              tunnel: inf -> [_ w390]
                              frame False {
                              }
                              frame True {
                              }
                            }
                            n420 = case shown="True" w376 {
                              tunnel: [u32 0 w392] -> w386
                              frame False {
                              }
                              frame True {
                                n421 = local read "Mark #"() -> (w394:u32)
                                n422 = local write "Trial #"(u32 0) -> ()
                                n423 = Increment(x=w394) -> (x+1=w392:u32)
                                n424 = local write "Mark #"(w392) -> ()
                              }
                            }
                            n425 = feedback #1() -> (w381:sgl)  [unwired: 1 in]
                            n426 = formula code="if(Tau==0) Tau=Tau+0.001;\nif(T==1) baselineflow=Tau;\n\ntmp=baselineflow/Tau;"("Tau"=w384, "T"=w388, "baselineflow"=w381) -> ("tmp"=w378:dbl, "baselineflow"=w382:sgl)
                            n427 = feedback-in #1(w382) -> ()
                            n428 = Bundle("tmp"=w378, w380) -> (→"Tau":cluster{"tmp":dbl, dbl})  [unwired: 1 in]
                          }
                          n429 = property on="Frame #" class="DigNum (strict)"() -> ("Value"=w322:u32)  [unwired: 2 in, 2 out]
                          n430 = case shown="True" "Fixed Time" {
                            tunnel: w322 -> [w364 w367]
                            tunnel: [w364 w367] -> w313
                            frame False {
                            }
                            frame True {
                              n431 = Less Or Equal?(x="Fixed # of Frames", y=w367) -> (x <= y?=w365:bool)
                              n432 = local write "Stop"(w365) -> ()
                            }
                          }
                          n433 = case shown="\"8 Detectors\", Default" w311 {
                            tunnel: w319 -> [w661 w665]
                            tunnel: [w662 w664] -> w348
                            tunnel: [4 8] -> w327
                            frame "4 Detectors" {
                              n434 = Build Array(w661, w661, w661, w661, w661) -> (w662:u32[])
                            }
                            frame "8 Detectors", Default {
                              n435 = Build Array(w665, w665, w665, w665, w665, w665, w665, w665, w665) -> (w664:u32[])
                            }
                          }
                          n436 = Increment(x=w313) -> (x+1=w323:u32)
                          n437 = local write "Frame #"(w323) -> ()
                          n438 = case shown="\"8 Detectors\", Default" w311 {
                            tunnel: ["%Duration\tID1\t\tID2\t\tID3\t\tID4\n" "%Duration\tID1\t\tID2\t\tID3\t\tID4\t\tID5\t\tID6\t\tID7\t\tID8\n"] -> w345
                            tunnel: ["%Tau\t\tTau1\t\tTau2\t\tTau3\t\tTau4\n" "%Tau\t\tTau1\t\tTau2\t\tTau3\t\tTau4\t\tTau5\t\tTau6\t\tTau7\t\tTau8\n"] -> w344
                            tunnel: ["%Delaytime\tD1\t\tD2\t\tD3\t\tD4\n" "%Delaytime\tD1\t\tD2\t\tD3\t\tD4\t\tD5\t\tD6\t\tD7\t\tD8\n"] -> w343
                            frame "4 Detectors" {
                            }
                            frame "8 Detectors", Default {
                            }
                          }
                          n439 = Number To Decimal String(number=w313) -> (decimal integer string=w349:string)  [unwired: 1 in]
                          n440 = Get Date/Time In Seconds() -> (seconds since 1Jan1904=w357:timestamp)
                          n441 = Array To Spreadsheet String(array=w348, 3:"%d") -> (spreadsheet string=w346:string)  [unwired: 1 in]
                          n442 = Format Date/Time String(seconds (now)=w357) -> (date/time string=w354:string)  [unwired: 2 in]
                          "Computer Time" <- w354
                          n443 = Concatenate Strings("File Name:", "_flow_", w349, ".dat") -> (w325:string)
                          n444 = Build Path(base path="Data Save Directory:", name or relative path=w325) -> (appended path=w317:path)
                          n445 = local read "Test"() -> (w321:bool)
                          n446 = Concatenate Strings("%", w354, "\r\n", w345, w342, w344, "%\t\t", w341, w343, w340, w346) -> (w329:string)
                          n447 = case shown="False" w321 {
                            tunnel: w329 -> [w361 _]
                            tunnel: w317 -> [w360 _]
                            tunnel: [w359 _] -> w316
                            tunnel: [w358 _] -> w315
                            frame False {
                              n448 = Write to Text File(file (use dialog)=w360, text=w361) -> (refnum out=w362:refnum<file>, error out=w363:errorcluster)  [unwired: 2 in, 1 out]
                              n449 = Close File(refnum=w362, error in=w363) -> (path=w359:path, error out=w358:errorcluster)
                            }
                            frame True {
                            }
                          }
                        }
                      }
                      n450 = local read "Test"() -> (w241:bool)
                      n451 = for {
                        N: 1 -> [_]
                        tunnel: w268 -> [_]
                        n452 = local write "Stop"(FALSE) -> ()
                        n453 = Wait (ms)(milliseconds to wait="Delay between frames(ms)") -> ()  [unwired: 1 out]
                      }
                      n454 = Unbundle By Name(w248) -> ("status"=w267:bool)
                      n455 = Not(x=w241) -> (.not. x?=w236:bool)
                      n456 = Not(x=w267) -> (.not. x?=w266:bool)
                      n457 = And(x="Real Time Fitting?", y=w236) -> (x .and. y?=w240:bool)
                      n458 = case shown="True" w240 {
                        tunnel: w266 -> [_ w275]
                        tunnel: w247 -> [_ w274]
                        tunnel: w246 -> [_ w273]
                        tunnel: w243 -> [w270 w272]
                        tunnel: [w270 w271] -> w242
                        frame False {
                        }
                        frame True {
                          n459 = case shown="True" w275 {
                            tunnel: w274 -> [_ w295]
                            tunnel: w273 -> [_ w291]
                            tunnel: w272 -> [w276 w287]
                            tunnel: [w276 w285] -> w271
                            frame False {
                            }
                            frame True {
                              # "Initialize Array of NaNs with size of \"fixed number of frames, \nand run this array into the case structure by putting it \nthrough a shift register with each loop it will replace one of \nthe NaNs by the flow data of the detector used. Then this data\nis averaged and COV is calculated."
                              n460 = property on="Data Save Directory:" class="Path"() -> ("Value"=w297:path)  [unwired: 2 in, 2 out]
                              n461 = property on="File Name:" class="Str"() -> ("Value"=w298:string)  [unwired: 2 in, 2 out]
                              n462 = call "GetFilePath.vi"("path"=w297, "file name"=w298, "frame number"=w295) -> ("final path C"=w290:string)  [unwired: 10 in, 2 out]
                              n463 = property on="Avg" class="Arr (strict)"() -> ("Value"=w296:bool[][])  [unwired: 2 in, 2 out]
                              n464 = call "DCSAnalysis.vi"("# Detectors"=w291, "File path"=w290, "Frame #"=w295, "rho"="rho", "other settings"="Other Settings", "avgBool"=w296, "var values"="Initial Guess") -> ("Flow in each detector"=w288:dbl[], "Tau"=→"Tau 2":T3)  [unwired: 18 in, 1 out]
                              "Flow in each detector" <- w288
                              n465 = local read "Detector Used"() -> (w278:T2)
                              n466 = local read "Trial #"() -> (w283:u32)
                              n467 = Decrement(x=w283) -> (x-1=w284:u32)
                              n468 = Index Array(array=w288, index=w278) -> (element=w286:dbl)
                              n469 = Replace Array Subset(array=w287, new element=w286, index=w284) -> (w285:dbl[])
                              n470 = call <vilib>:"Std Deviation and Variance.vi"("X"=w285) -> ("mean"=w281:dbl, "standard deviation"=w282:dbl)  [unwired: 1 in, 1 out]
                              "mean" <- w281
                              n471 = Divide(x=w282, y=w281) -> (x/y=w280:dbl)
                              n472 = Multiply(x=w280, y=100.0) -> (x*y=→"COV":dbl)
                            }
                          }
                        }
                      }
                    }
                    n473 = call "iBs.vi"("Laser On/Off"=TRUE, "VISA resource name"="Laser Input Name") -> ()
                    n474 = Build Array(FALSE) -> (w222:bool[])
                    n475 = call "DAQ Assistant7"("data"=w222) -> ()  [unwired: 17 in, 2 out]
                    n476 = local read "Test"() -> (w216:bool)
                    n477 = case shown="False" w216 {
                      frame False {
                        # "This bit stores the time stamp."
                        n478 = local read "File Name:"() -> (w226:string)
                        n479 = Get Date/Time In Seconds() -> (seconds since 1Jan1904=w228:timestamp)
                        n480 = local read "Data Save Directory:"() -> (w227:path)
                        n481 = Format Date/Time String(seconds (now)=w228) -> (date/time string=w234:string)  [unwired: 2 in]
                        n482 = Concatenate Strings(w226, "_TIMING", ".dat") -> (w231:string)
                        n483 = Build Path(base path=w227, name or relative path=w231) -> (appended path=w230:path)
                        n484 = Write to Text File(file (use dialog)=w230, text=w234) -> (refnum out=w233:refnum<file>, error out=w232:errorcluster)  [unwired: 2 in, 1 out]
                        n485 = Close File(refnum=w233, error in=w232) -> ()  [unwired: 2 out]
                      }
                      frame True {
                      }
                    }
                  }
                  frame True {
                    n486 = invoke on="Sequence Scan" class="Bool" method="Reinit To Default"() -> ()  [unwired: 3 in, 3 out]
                    n487 = call "Display Message to User5"() -> ()  [unwired: 10 in, 2 out]
                  }
                }
              }
            }
            "Frame #" <- u32 0
            "Mark #" <- u32 0
            "Trial #" <- u32 0
          }
          event "QUIT": Value Change {
            # "Reset correlator before quitting"
            n488 = event-data() -> ()  [unwired: 1 in, 6 out]
            n489 = local write "Status"("Quit") -> ()
            n490 = case shown="\"8 Detectors\", Default" w674 {
              frame "4 Detectors" {
                n491 = dll-call lib="C:/Users/BUCKLEY-ADMIN/Desktop/DCScode_simulISS_MAP/flex05-4chPascal.dll" fn="USBInitialize" label="InitCH4"() -> (error out=w675:errorcluster)  [unwired: 4 in, 1 out]
                n492 = dll-call lib="C:/Users/BUCKLEY-ADMIN/Desktop/DCScode_simulISS_MAP/flex05-4chPascal.dll" fn="USBFree" label="FreeCH4"(error in=w675) -> ()  [unwired: 3 in, 2 out]
              }
              frame "8 Detectors", Default {
                n493 = dll-call lib="C:/Users/BUCKLEY-ADMIN/Desktop/DCScode_simulISS_MAP/flex05oem8chauto100nsPASCAL_win7.dll" fn="USBInitialize" label="InitCH8"() -> (error out=w676:errorcluster)  [unwired: 4 in, 1 out]
                n494 = dll-call lib="C:/Users/BUCKLEY-ADMIN/Desktop/DCScode_simulISS_MAP/flex05oem8chauto100nsPASCAL_win7.dll" fn="USBFree" label="FreeCH8"(error in=w676) -> ()  [unwired: 3 in, 2 out]
              }
            }
            n495 = local write "Status"("Quit") -> ()
          }
          event Timeout {
            w681 = TRUE
            w680 = u8 0
            # "This case structure turns on\n      and off the ISS Lasers"
            # "This case structure ensures that when the\noptical switch is turned on, the relay tells \nthe laser to power on."
            # "The system sits here and wait for some buttons to be pressed. And the status is always \"waiting\". Once some button is pressed, this value driven event\nstructure goes to the appropriate frame."
            n496 = event-data() -> ()  [unwired: 1 in, 3 out]
            n497 = local write "Status"("Waiting") -> ()
            n498 = property on="MARK\nMark" class="Bool"("DisabledEnum"=w680) -> ()  [unwired: 2 in, 2 out]
            n499 = property on="QUIT" class="Bool (strict)"("Disabled"=w680) -> ()  [unwired: 2 in, 2 out]
            n500 = property on="Sequence Scan" class="Bool"("Disabled"=w680) -> ()  [unwired: 2 in, 2 out]
            n501 = property on="Initialize Correlator" class="Bool"("Disabled"=w680) -> ()  [unwired: 2 in, 2 out]
            n502 = property on="Update Time (ms)\nDO NOT CHANGE!" class="DigNum (strict)"("Disabled"=w680) -> ()  [unwired: 2 in, 2 out]
            n503 = property on="Integration Time (ms)" class="DigNum (strict)"("Disabled"=w680) -> ()  [unwired: 2 in, 2 out]
            n504 = property on="Detector Select" class="RadioBtnsControl (strict)"("Disabled"=w680) -> ()  [unwired: 2 in, 2 out]
            n505 = case shown="True" "ISS Lasers ON" {
              frame False {
                n506 = Build Array(FALSE) -> (w688:bool[])
                n507 = call "DAQ Assistant5"("data"=w688) -> ()  [unwired: 17 in, 2 out]
              }
              frame True {
                # "For Toptica laser control"
                n508 = local read "Laser Input Name"() -> (w690:refnum<visa-resource-name>)
                n509 = call "iBs.vi"("Laser On/Off"=TRUE, "VISA resource name"=w690) -> ()
                n510 = Build Array(TRUE) -> (w692:bool[])
                n511 = call "DAQ Assistant6"("data"=w692) -> ()  [unwired: 17 in, 2 out]
              }
            }
            n512 = case shown="True" "Optical Switch OPEN" {
              frame False {
                # "Send 2 signals, one for LED indicator, one for switch"
                n513 = Build Array(FALSE, FALSE) -> (w694:bool[])
                n514 = call "DAQ Assistant3"("data"=w694) -> ()  [unwired: 17 in, 2 out]
              }
              frame True {
                n515 = Build Array(TRUE, TRUE) -> (w697:bool[])
                n516 = call "DAQ Assistant4"("data"=w697) -> ()  [unwired: 17 in, 2 out]
              }
            }
            n517 = Current VI's Menubar() -> (w683:refnum<k9>)
            n518 = Set Menu Item Info(7:"File", 9:w681, 11:w683) -> (3:w682:refnum<k9>)  [unwired: 4 in, 1 out]
            n519 = Get Date/Time In Seconds() -> (seconds since 1Jan1904=w686:timestamp)
            n520 = Set Menu Item Info(7:"Options", 9:w681, 11:w682) -> ()  [unwired: 4 in, 2 out]
            n521 = Format Date/Time String(seconds (now)=w686) -> (date/time string=w687:string)  [unwired: 2 in]
            n522 = local write "Computer Time"(w687) -> ()
          }
        }
      }
    }
  }
  "Trial In Progress" <- FALSE ("Trial In Progress")
